vi "Periodic Tasks.vi"(8 "error in":errorcluster) -> (0 "error out":errorcluster)   [LabVIEW 2018]
doc: "This VI runs in parallel to other tasks. It can contain as many user-defined periodic loops as you need. These can carry out PID or other sorts of timed response."
uses:
  <vilib>/Rock Robotics/WPI/Joystick/WPI_JoystickDevRef.ctl
  <vilib>/Rock Robotics/WPI/Joystick/WPI_JoystickDeviceEnum.ctl
  <vilib>/Rock Robotics/WPI/RobotDrive/WPI_RobotDriveDevRef.ctl
  <vilib>/Rock Robotics/WPI/MotorControl/WPI_MotorControlDeviceRef.ctl
  <vilib>/Rock Robotics/WPI/MotorControl/WPI_MotorControlType.ctl
  <vilib>/Rock Robotics/SystemInterfaces/DIO/FPGA_DIOPWMChannel.ctl
  <vilib>/Rock Robotics/WPI/PWM/WPI_PWMDeadband.ctl
  <vilib>/Rock Robotics/SystemInterfaces/DIO/FPGA_DIOChannel.ctl
  <vilib>/Rock Robotics/WPI/Solenoid/WPI_SolenoidDevRef.ctl
  <vilib>/Rock Robotics/WPI/Solenoid/WPI_SolenoidChannel.ctl
  <vilib>/Rock Robotics/WPI/DigitalInput/WPI_DigitalInputDevRef.ctl
  Vision States.ctl
  <vilib>/Rock Robotics/WPI/DriverStation/WPI_DriverStationRobotMode2.ctl
  Hatch Retainer States.ctl
  HAB Bk Spd Motor States.ctl
  <vilib>/Rock Robotics/WPI/Solenoid/WPI_SolenoidValue.ctl
  <vilib>/Rock Robotics/WPI/ThirdParty/Phoenix-LabVIEW/Motor Controller/Controls/CTRE_Phoenix_MotorControl_ControlMode.ctl
  <vilib>/Rock Robotics/WPI/ThirdParty/Phoenix-LabVIEW/Motor Controller/Controls/CTRE_Phoenix_MotorControl_MotionProfileTrajectoryPoint.ctl
  <vilib>/Rock Robotics/WPI/Utilities/WPI_GetSetVariantRefNum.vi
  <vilib>/Rock Robotics/WPI/ThirdParty/Phoenix-LabVIEW/Motor Controller/Get/CTRE_Phoenix_MotorController_GetQuadratureData.vi
  Robot Global Data.vi
  <vilib>/addons/control/pid/pid.llb/PID (DBL).vi
  <vilib>/Rock Robotics/WPI/Solenoid/WPI_SolenoidSetEnum.vi
  <vilib>/Rock Robotics/Network Tables/NT Write Number.vi
  <vilib>/Rock Robotics/WPI/ThirdParty/Phoenix-LabVIEW/Motor Controller/Closed Loop/Motion Profile/CTRE_Phoenix_MotorControl_BufferedTrajectoryPointStream_WriteAll.vi
  <vilib>/Rock Robotics/Network Tables/NT Read Number.vi
  <vilib>/addons/control/pid/NI_PID_pid.lvlib
panel:
  in  "BkSpdAdjusterMotorDevRef":T1={"DeviceStatus"={"status"=FALSE, "code"=0, "source"=""}, "Type"=enum."PWM", "PWM"={"PWM Channel"=enum."Invalid", "DeadBand"={"Name"="", "maxPositivePwm"=0, "minPositivePwm"=0, "centerPwm"=0, "maxNegativePwm"=0, "minNegativePwm"=0, "angularRange"=0}}, "CAN"={"Device Number"=0, "SetOutput VI Ref"=variant(refnum<vi> refnum), "GetOutput VI Ref"=variant(refnum<vi> refnum), "Enable VI Ref"=variant(refnum<vi> refnum), "Disable VI Ref"=variant(refnum<vi> refnum), "Data"=variant}, "Invert"=FALSE, "DIO PWM"={"PWM \"Enable\" Channel"=enum."Invalid", "DIOChannel"=enum."Invalid", "PWM Rate"=0.0}}
  in  "HABAssisterSolenoidDevRef":T6={"DevStatus"={"status"=FALSE, "code"=0, "source"=""}, "Pneumatics Control Module"=0, "Forward Solenoid Channel"=enum."Invalid", "Reverse Solenoid Channel"=enum."Invalid"}
  out "Right Traj. Pts Array":dbl[][](array[numeric])
  out "Left Traj. Pts Array":dbl[][](array[numeric])
  in  "Back HAB 3 Limit Switch":T8={"DevStatus"={"status"=FALSE, "code"=0, "source"=""}, "DIO Channel"=enum."Invalid"}
  in  "Front HAB 3 Limit Switch":T8={"DevStatus"={"status"=FALSE, "code"=0, "source"=""}, "DIO Channel"=enum."Invalid"}
  in  "BottomRetainerSwitchDevRef":T8={"DevStatus"={"status"=FALSE, "code"=0, "source"=""}, "DIO Channel"=enum."Invalid"}
  in  "TopRetainerSwitchDevRef":T8={"DevStatus"={"status"=FALSE, "code"=0, "source"=""}, "DIO Channel"=enum."Invalid"}
  in  "HatchRetainerMotorDevRef":T1={"DeviceStatus"={"status"=FALSE, "code"=0, "source"=""}, "Type"=enum."PWM", "PWM"={"PWM Channel"=enum."Invalid", "DeadBand"={"Name"="", "maxPositivePwm"=0, "minPositivePwm"=0, "centerPwm"=0, "maxNegativePwm"=0, "minNegativePwm"=0, "angularRange"=0}}, "CAN"={"Device Number"=0, "SetOutput VI Ref"=variant(refnum<vi> refnum), "GetOutput VI Ref"=variant(refnum<vi> refnum), "Enable VI Ref"=variant(refnum<vi> refnum), "Disable VI Ref"=variant(refnum<vi> refnum), "Data"=variant}, "Invert"=FALSE, "DIO PWM"={"PWM \"Enable\" Channel"=enum."Invalid", "DIOChannel"=enum."Invalid", "PWM Rate"=0.0}}
  in  "HAB3BackSolenoidDevRef":T6={"DevStatus"={"status"=FALSE, "code"=0, "source"=""}, "Pneumatics Control Module"=0, "Forward Solenoid Channel"=enum."Invalid", "Reverse Solenoid Channel"=enum."Invalid"}
  in  "HAB3FrontSolenoidDevRef":T6={"DevStatus"={"status"=FALSE, "code"=0, "source"=""}, "Pneumatics Control Module"=0, "Forward Solenoid Channel"=enum."Invalid", "Reverse Solenoid Channel"=enum."Invalid"}
  in  "AuxJoystickDevRef":T9={"Device"=enum."USB 1"}
  in  "DriveJoystickDevRef":T9={"Device"=enum."USB 1"}
  in  "HAB3DriveModuleMotorDevRef":T1={"DeviceStatus"={"status"=FALSE, "code"=0, "source"=""}, "Type"=enum."PWM", "PWM"={"PWM Channel"=enum."Invalid", "DeadBand"={"Name"="", "maxPositivePwm"=0, "minPositivePwm"=0, "centerPwm"=0, "maxNegativePwm"=0, "minNegativePwm"=0, "angularRange"=0}}, "CAN"={"Device Number"=0, "SetOutput VI Ref"=variant(refnum<vi> refnum), "GetOutput VI Ref"=variant(refnum<vi> refnum), "Enable VI Ref"=variant(refnum<vi> refnum), "Disable VI Ref"=variant(refnum<vi> refnum), "Data"=variant}, "Invert"=FALSE, "DIO PWM"={"PWM \"Enable\" Channel"=enum."Invalid", "DIOChannel"=enum."Invalid", "PWM Rate"=0.0}}
  in  "LifterSolenoidDevRef":T6={"DevStatus"={"status"=FALSE, "code"=0, "source"=""}, "Pneumatics Control Module"=0, "Forward Solenoid Channel"=enum."Invalid", "Reverse Solenoid Channel"=enum."Invalid"}
  in  "DriveJoystickDevRef":T9={"Device"=enum."USB 1"}
  in  "HatchCollectorMotorDevRef":T1={"DeviceStatus"={"status"=FALSE, "code"=0, "source"=""}, "Type"=enum."PWM", "PWM"={"PWM Channel"=enum."Invalid", "DeadBand"={"Name"="", "maxPositivePwm"=0, "minPositivePwm"=0, "centerPwm"=0, "maxNegativePwm"=0, "minNegativePwm"=0, "angularRange"=0}}, "CAN"={"Device Number"=0, "SetOutput VI Ref"=variant(refnum<vi> refnum), "GetOutput VI Ref"=variant(refnum<vi> refnum), "Enable VI Ref"=variant(refnum<vi> refnum), "Disable VI Ref"=variant(refnum<vi> refnum), "Data"=variant}, "Invert"=FALSE, "DIO PWM"={"PWM \"Enable\" Channel"=enum."Invalid", "DIOChannel"=enum."Invalid", "PWM Rate"=0.0}}
  in  "AuxJoystickDevRef":T9
  in  "RetainerSolenoidDevRef":T6={"DevStatus"={"status"=FALSE, "code"=0, "source"=""}, "Pneumatics Control Module"=0, "Forward Solenoid Channel"=enum."Invalid", "Reverse Solenoid Channel"=enum."Invalid"}
  in  "KickerSolenoidDevRef":T6={"DevStatus"={"status"=FALSE, "code"=0, "source"=""}, "Pneumatics Control Module"=0, "Forward Solenoid Channel"=enum."Invalid", "Reverse Solenoid Channel"=enum."Invalid"}
  in  "Drive Motors":T11={"DevStatus"={"status"=FALSE, "code"=0, "source"=""}, "Motors[]"=[], "Square Inputs"=FALSE, "Max Output"=1.0}
  in  "AuxJoystickDevRef":T9={"Device"=enum."USB 1"}
  in  "DriveJoystickDevRef":T9
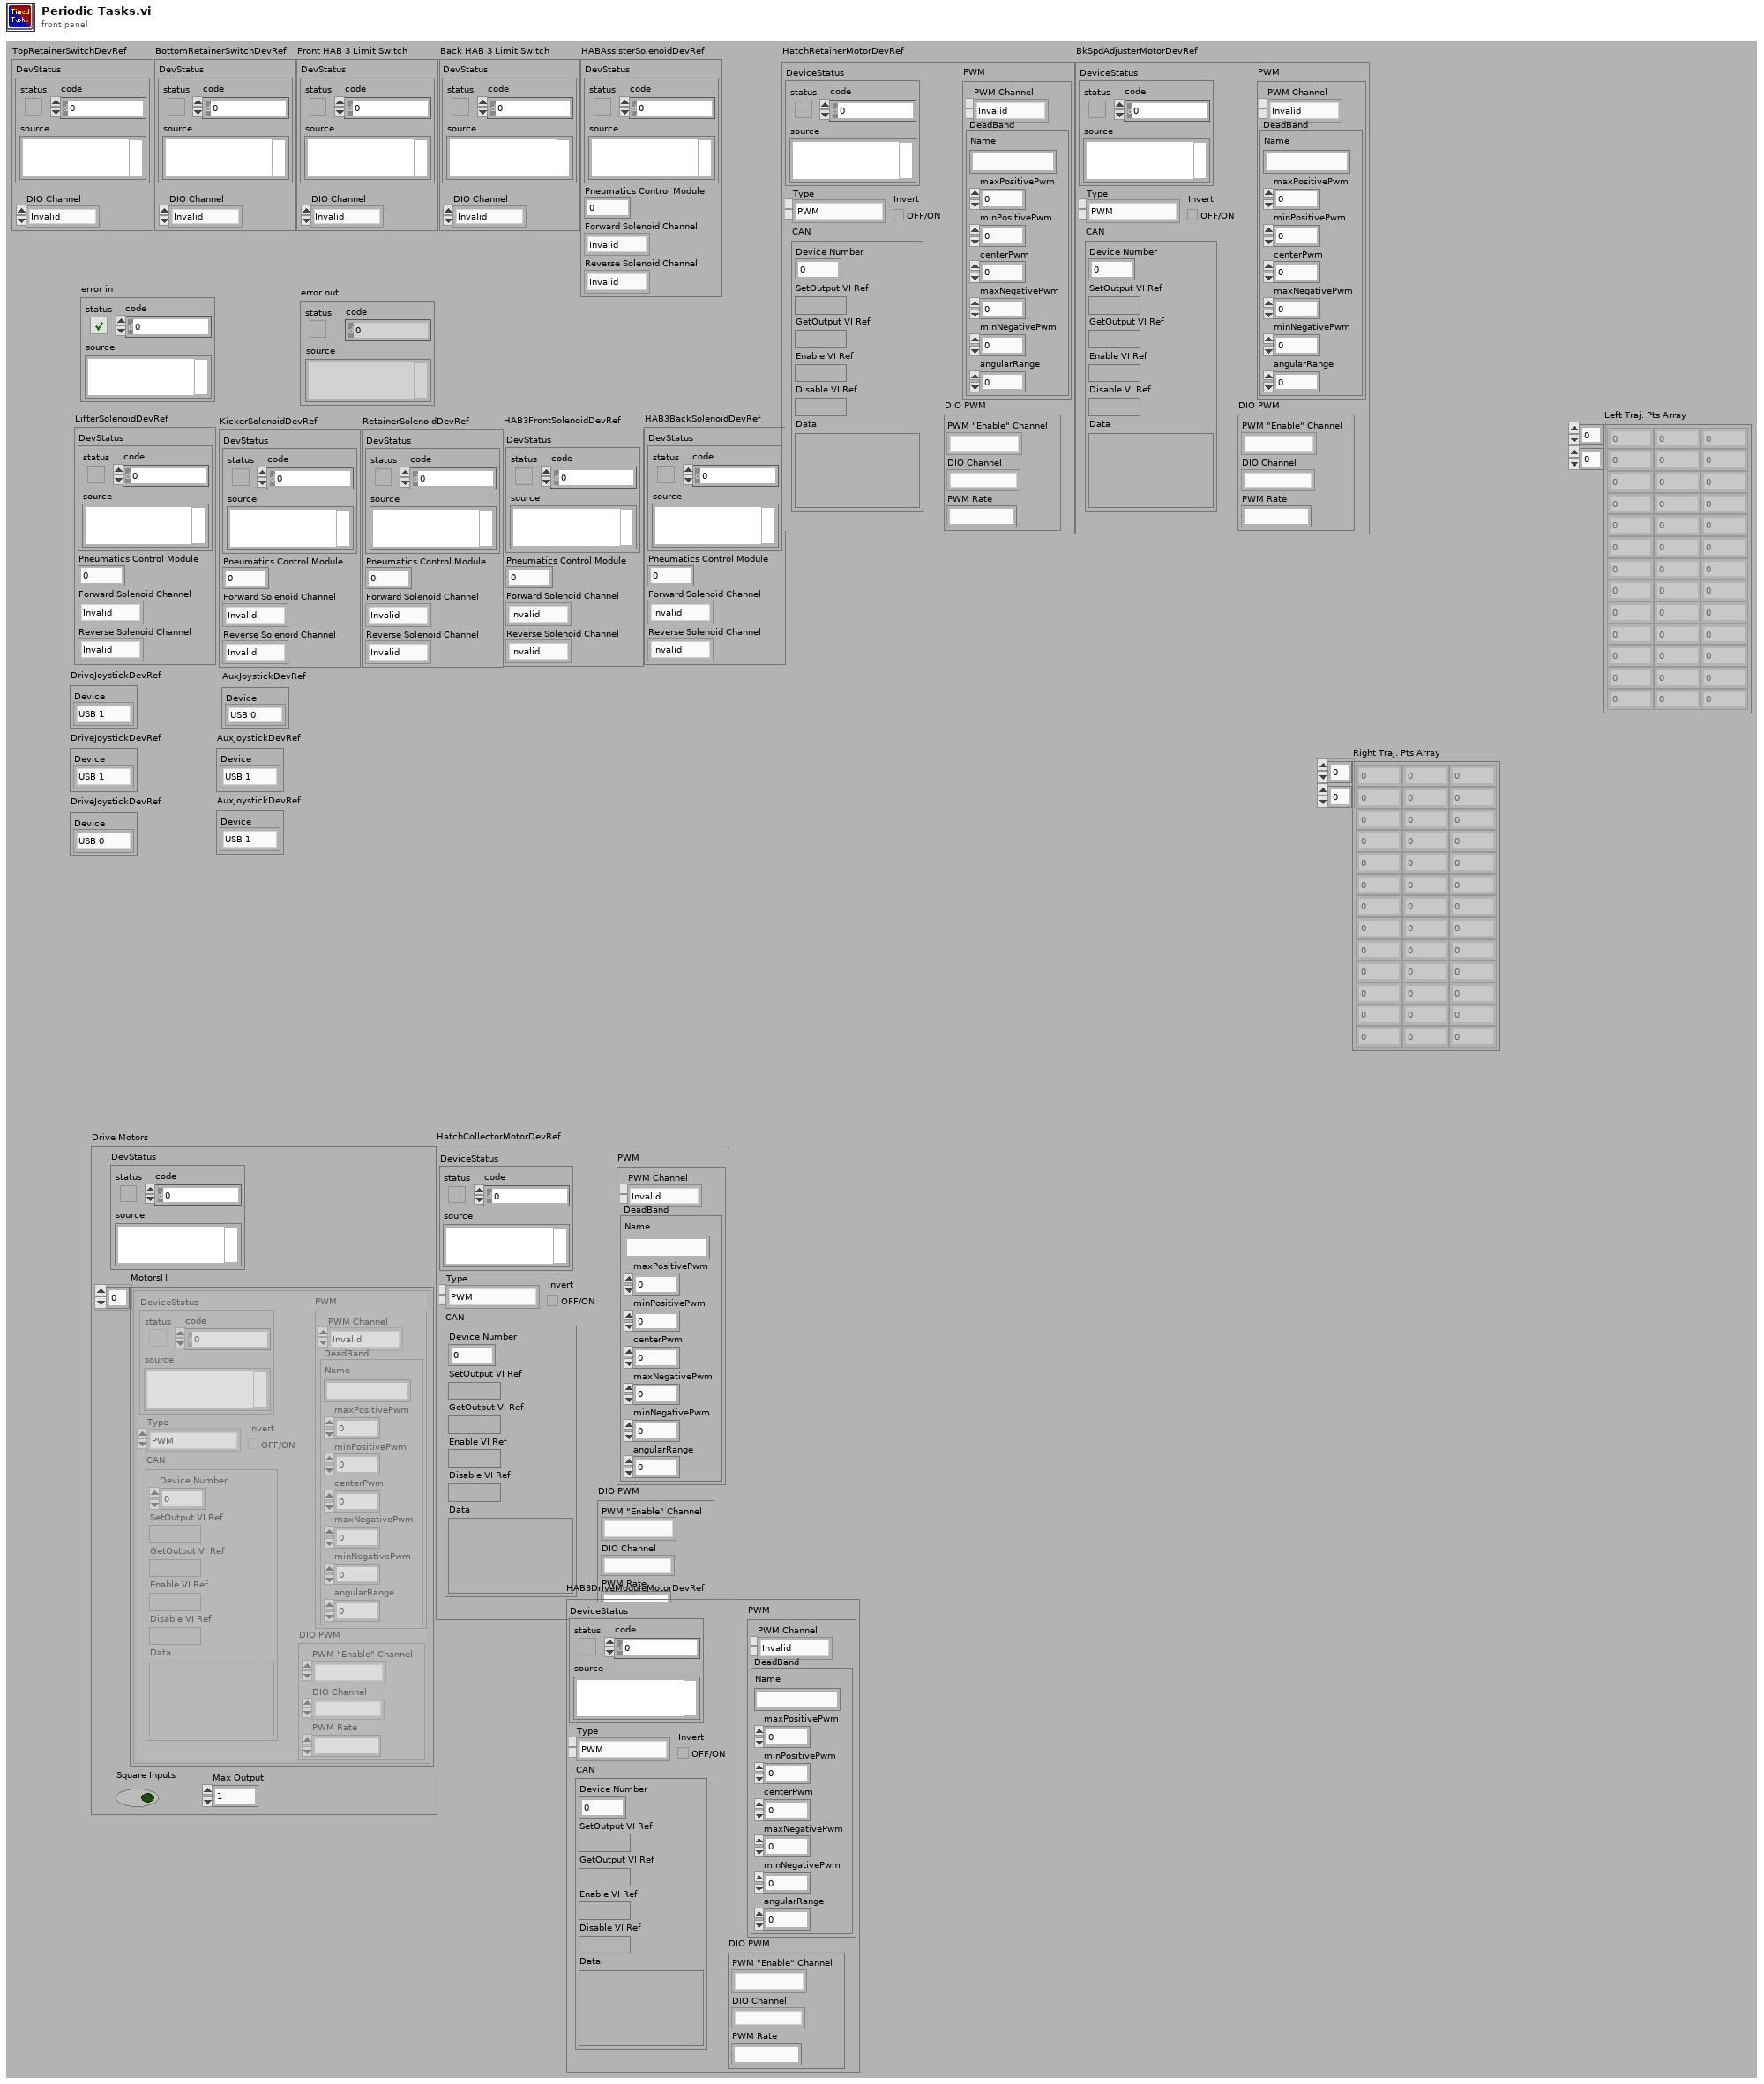
[diagram p1: front panel]
types:
  T1 = typedef "WPI_MotorControlDeviceRef.ctl" = cluster{"DeviceStatus":errorcluster, "Type":T2, "PWM":cluster{"PWM Channel":T3, "DeadBand":T4}, "CAN":cluster{"Device Number":u8, "SetOutput VI Ref":variant, "GetOutput VI Ref":variant, "Enable VI Ref":variant, "Disable VI Ref":variant, "Data":variant}, "Invert":bool, "DIO PWM":cluster{"PWM \"Enable\" Channel":T3, "DIOChannel":T5, "PWM Rate":dbl}}
  T2 = typedef "WPI_MotorControlType.ctl" = enum16{"PWM", "CAN", "DIO PWM"}
  T3 = typedef "FPGA_DIOPWMChannel.ctl" = enum8{"PWM 0", "PWM 1", "PWM 2", "PWM 3", "PWM 4", "PWM 5", "PWM 6", "PWM 7", "PWM 8", "PWM 9", "PWM MXP 0", "PWM MXP 1", "PWM MXP 2", "PWM MXP 3", "PWM MXP 4", "PWM MXP 5", "PWM MXP 6", "PWM MXP 7", "PWM MXP 8", "PWM MXP 9", "Invalid"}
  T4 = typedef "WPI_PWMDeadband.ctl" = cluster{"Name":string, "maxPositivePwm":i32, "minPositivePwm":i32, "centerPwm":i32, "maxNegativePwm":i32, "minNegativePwm":i32, "angularRange":u16}
  T5 = typedef "FPGA_DIOChannel.ctl" = enum8{"DIO 0", "DIO 1", "DIO 2", "DIO 3", "DIO 4", "DIO 5", "DIO 6", "DIO 7", "DIO 8", "DIO 9", "DIO MXP 0", "DIO MXP 1", "DIO MXP 2", "DIO MXP 3", "DIO MXP 4", "DIO MXP 5", "DIO MXP 6", "DIO MXP 7", "DIO MXP 8", "DIO MXP 9", "DIO MXP 10", "DIO MXP 11", "DIO MXP 12", "DIO MXP 13", "DIO MXP 14", "DIO MXP 15", "SPI Port CS1", "SPI Port CS2", "SPI Port CS3", "SPI Port MISO", "SPI Port MOSI", "Invalid"}
  T6 = typedef "WPI_SolenoidDevRef.ctl" = cluster{"DevStatus":errorcluster, "Pneumatics Control Module":u8, "Forward Solenoid Channel":T7, "Reverse Solenoid Channel":T7}
  T7 = typedef "WPI_SolenoidChannel.ctl" = enum8{"Solenoid 0", "Solenoid 1", "Solenoid 2", "Solenoid 3", "Solenoid 4", "Solenoid 5", "Solenoid 6", "Solenoid 7", "Invalid"}
  T8 = typedef "WPI_DigitalInputDevRef.ctl" = cluster{"DevStatus":errorcluster, "DIO Channel":T5}
  T9 = typedef "WPI_JoystickDevRef.ctl" = cluster{"Device":T10}
  T10 = typedef "WPI_JoystickDeviceEnum.ctl" = enum16{"USB 0", "USB 1", "USB 2", "USB 3", "USB 4", "USB 5"}
  T11 = typedef "WPI_RobotDriveDevRef.ctl" = cluster{"DevStatus":errorcluster, "Motors[]":T1[], "Square Inputs":bool, "Max Output":dbl}
  T12 = typedef "HAB Bk Spd Motor States.ctl" = enum16{"Fully Up", "Going Down", "Fully Down", "Going Up"}
  T13 = typedef "Hatch Retainer States.ctl" = enum16{"Fully Down", "Going Up", "Fully Up", "Going Down"}
  T14 = cluster{"X Button":i32, "A Button":i32, "B Button":i32, "Y Button":i32, "LB Button":i32, "RB Button":i32, "LT Button":i32, "RT Button":i32, "BACK Button":i32, "START Button":i32, "LJ Click Button":i32, "RJ Click Button":i32}
  T15 = cluster{"Left X":i32, "Left Y":i32, "Right X":i32, "Right Y":i32}
  T16 = typedef "WPI_DriverStationRobotMode2.ctl" = enum16{"Autonomous Disabled", "Autonomous Enabled", "Teleop Disabled", "Teleop Enabled", "Disconnected", "Finish", "Test Disabled", "Test Enabled", "Emergency Stopped"}
  T17 = cluster{"offsetAngle H":dbl, "offsetAngle V":dbl, "area":dbl, "skew":dbl, "shortest side (pxls)":dbl, "longest side (pxls)":dbl}
  T18 = typedef "Vision States.ctl" = enum16{"Ready", "Forward Until Target at Edge", "Vision Track"}
  T19 = cluster{"A Button":i32, "B Button":i32, "X Button":i32, "Y Button":i32, "LB Button":i32, "RB Button":i32, "BACK Button":i32, "START Button":i32, "LJ Click Button":i32, "RJ Click Button":i32}
  T20 = typedef "WPI_GyroDevRef.ctl" = cluster{"DevStatus":errorcluster, "Analog Channel":T21, "Gain (VoltsPerDegree/Second)":dbl, "Gyro Type":enum16{"Analog", "XRS450"}, "Handle":i32, "SPI Bus":T22, "Device Found":bool, "Sample Rate":dbl, "Calibrate On Open":bool, "Offset":dbl}
  T21 = typedef "FPGA_AIChannel.ctl" = enum8{"AI 0", "AI 1", "AI 2", "AI 3", "AI MXP 0", "AI MXP 1", "AI MXP 2", "AI MXP 3", "Invalid"}
  T22 = typedef "spi_bus.ctl" = enum16{"SPI On-Board, CS0", "SPI On-Board, CS1", "SPI On-Board, CS2", "SPI On-Board, CS3", "SPI MXP", "Invalid"}
  T23 = cluster{"DriveJoystickDevRef":T9, "AuxJoystickDevRef":T9, "Drive Axes":dbl[], "Drive Buttons":bool[], "Drive POVs":i16[], "Aux Axes":dbl[], "Aux Buttons":bool[], "Aux POVs":i16[], "Robot Mode":T16, "Drive Motors":T11, "Drive Joystick Indexes":cluster{"Left X":i32, "Left Y":i32, "Right X":i32, "Right Y":i32}, "Drive Button Indexes":cluster{"A Button":i32, "B Button":i32, "X Button":i32, "Y Button":i32, "LB Button":i32, "RB Button":i32, "BACK Button":i32, "START Button":i32, "LJ Click Button":i32, "RJ Click Button":i32}, "Joystick VS Vision Latch":bool, "Vision States":T18, "limelight":cluster{"offsetAngle H":dbl, "offsetAngle V":dbl, "area":dbl, "skew":dbl, "shortest side (pxls)":dbl, "longest side (pxls)":dbl}, "Vision Track Mode Override":bool, "T = Motion Profile, F = Percent Output":bool}
  T24 = cluster{"TopRetainerSwitchDevRef":T8, "BottomRetainerSwitchDevRef":T8, "HatchRetainerMotorDevRef":T1, "LifterSolenoidDevRef":T6, "DriveJoystickDevRef":T9, "KickerSolenoidDevRef":T6, "RetainerSolenoidDevRef":T6, "AuxJoystickDevRef":T9, "HatchCollectorMotorDevRef":T1, "Drive Axes":dbl[], "Drive Buttons":bool[], "Drive POVs":i16[], "Aux Axes":dbl[], "Aux Buttons":bool[], "Aux POVs":i16[], "Robot Mode":T16, "Aux Joystick Indexes":cluster{"Left X":i32, "Left Y":i32, "Right X":i32, "Right Y":i32}, "Aux Button Indexes":cluster{"X Button":i32, "A Button":i32, "B Button":i32, "Y Button":i32, "LB Button":i32, "RB Button":i32, "LT Button":i32, "RT Button":i32, "BACK Button":i32, "START Button":i32, "LJ Click Button":i32, "RJ Click Button":i32}, "Hatch Retainer Move Up/Down":bool, "Hatch Collector Actual Angle":dbl, "Hatch Collector Wanted Angle":dbl, "Hatch Retainer States":T13}
  T25 = cluster{"BkSpdAdjusterMotorDevRef":T1, "HABAssisterSolenoidDevRef":T6, "Back HAB 3 Limit Switch":T8, "Front HAB 3 Limit Switch":T8, "HAB3DriveModuleMotorDevRef":T1, "DriveJoystickDevRef":T9, "AuxJoystickDevRef":T9, "HAB3FrontSolenoidDevRef":T6, "HAB3BackSolenoidDevRef":T6, "Drive Axes":dbl[], "Drive Buttons":bool[], "Drive POVs":i16[], "Aux Axes":dbl[], "Aux Buttons":bool[], "Aux POVs":i16[], "Robot Mode":T16, "Aux Joystick Indexes":cluster{"Left X":i32, "Left Y":i32, "Right X":i32, "Right Y":i32}, "Aux Button Indexes":cluster{"X Button":i32, "A Button":i32, "B Button":i32, "Y Button":i32, "LB Button":i32, "RB Button":i32, "LT Button":i32, "RT Button":i32, "BACK Button":i32, "START Button":i32, "LJ Click Button":i32, "RJ Click Button":i32}, "Front Cylinders Latch":bool, "Back Cylinders Latch":bool, "Yaw":dbl, "Pitch":dbl, "Roll":dbl, "HAB Bk Spd Motor States":T12}
  T26 = typedef "WPI_SolenoidValue.ctl" = enum16{"Off", "On", "Forward", "Reverse"}
  T27 = cluster{"proportional gain (Kc)":dbl, "integral time (Ti, min)":dbl, "derivative time (Td, min)":dbl}
  T28 = typedef "Which Robot Enum.ctl" = enum16{"Competition Bot", "Practice Bot", "Code Bot"}
  T29 = typedef "CTRE_Phoenix_MotorControl_ControlMode.ctl" = u16
  T30 = cluster{"Yaw":dbl, "Roll":dbl, "Pitch":dbl, "Heading":dbl, "Fused Heading":dbl}
  T31 = typedef "CTRE_Phoenix_MotorControl_MotionProfileTrajectoryPoint.ctl" = cluster{"Position":dbl, "Velocity":dbl, "Arbitrary Feed Forward":dbl, "Auxiliary Position":dbl, "Auxiliary Velocity":dbl, "Auxiliary Arbitrary Feed Forward":dbl, "Profile Slot Select":i32, "Auxiliary Profile Slot Select":i32, "isLastPoint?":bool, "Zero Position?":bool, "durationMs":u32, "Use Aux PID?":bool}
  T32 = typedef "CTRE_Phoenix_MotorControl_BufferedTrajectoryPointStream_DeviceRef.ctl" = cluster{"Handle":u64, "Library Path":path}
  T33 = cluster{"DriveJoystickDevRef":T9, "AuxJoystickDevRef":T9, "Drive Axes":dbl[], "Drive Buttons":bool[], "Drive POVs":i16[], "Aux Axes":dbl[], "Aux Buttons":bool[], "Aux POVs":i16[], "Robot Mode":T16, "Drive Motors":T11, "Drive Joystick Indexes":cluster{"Left X":i32, "Left Y":i32, "Right X":i32, "Right Y":i32}, "Drive Button Indexes":cluster{"A Button":i32, "B Button":i32, "X Button":i32, "Y Button":i32, "LB Button":i32, "RB Button":i32, "BACK Button":i32, "START Button":i32, "LJ Click Button":i32, "RJ Click Button":i32}, "Joystick VS Vision Latch":bool, "Vision States":T18, "limelight":cluster{"offsetAngle H":dbl, "offsetAngle V":dbl, "area":dbl, "skew":dbl, "shortest side (pxls)":dbl, "longest side (pxls)":dbl}, "Vision Track Mode Override":bool, "T = Motion Profile, F = Percent Output (Latch)":bool}
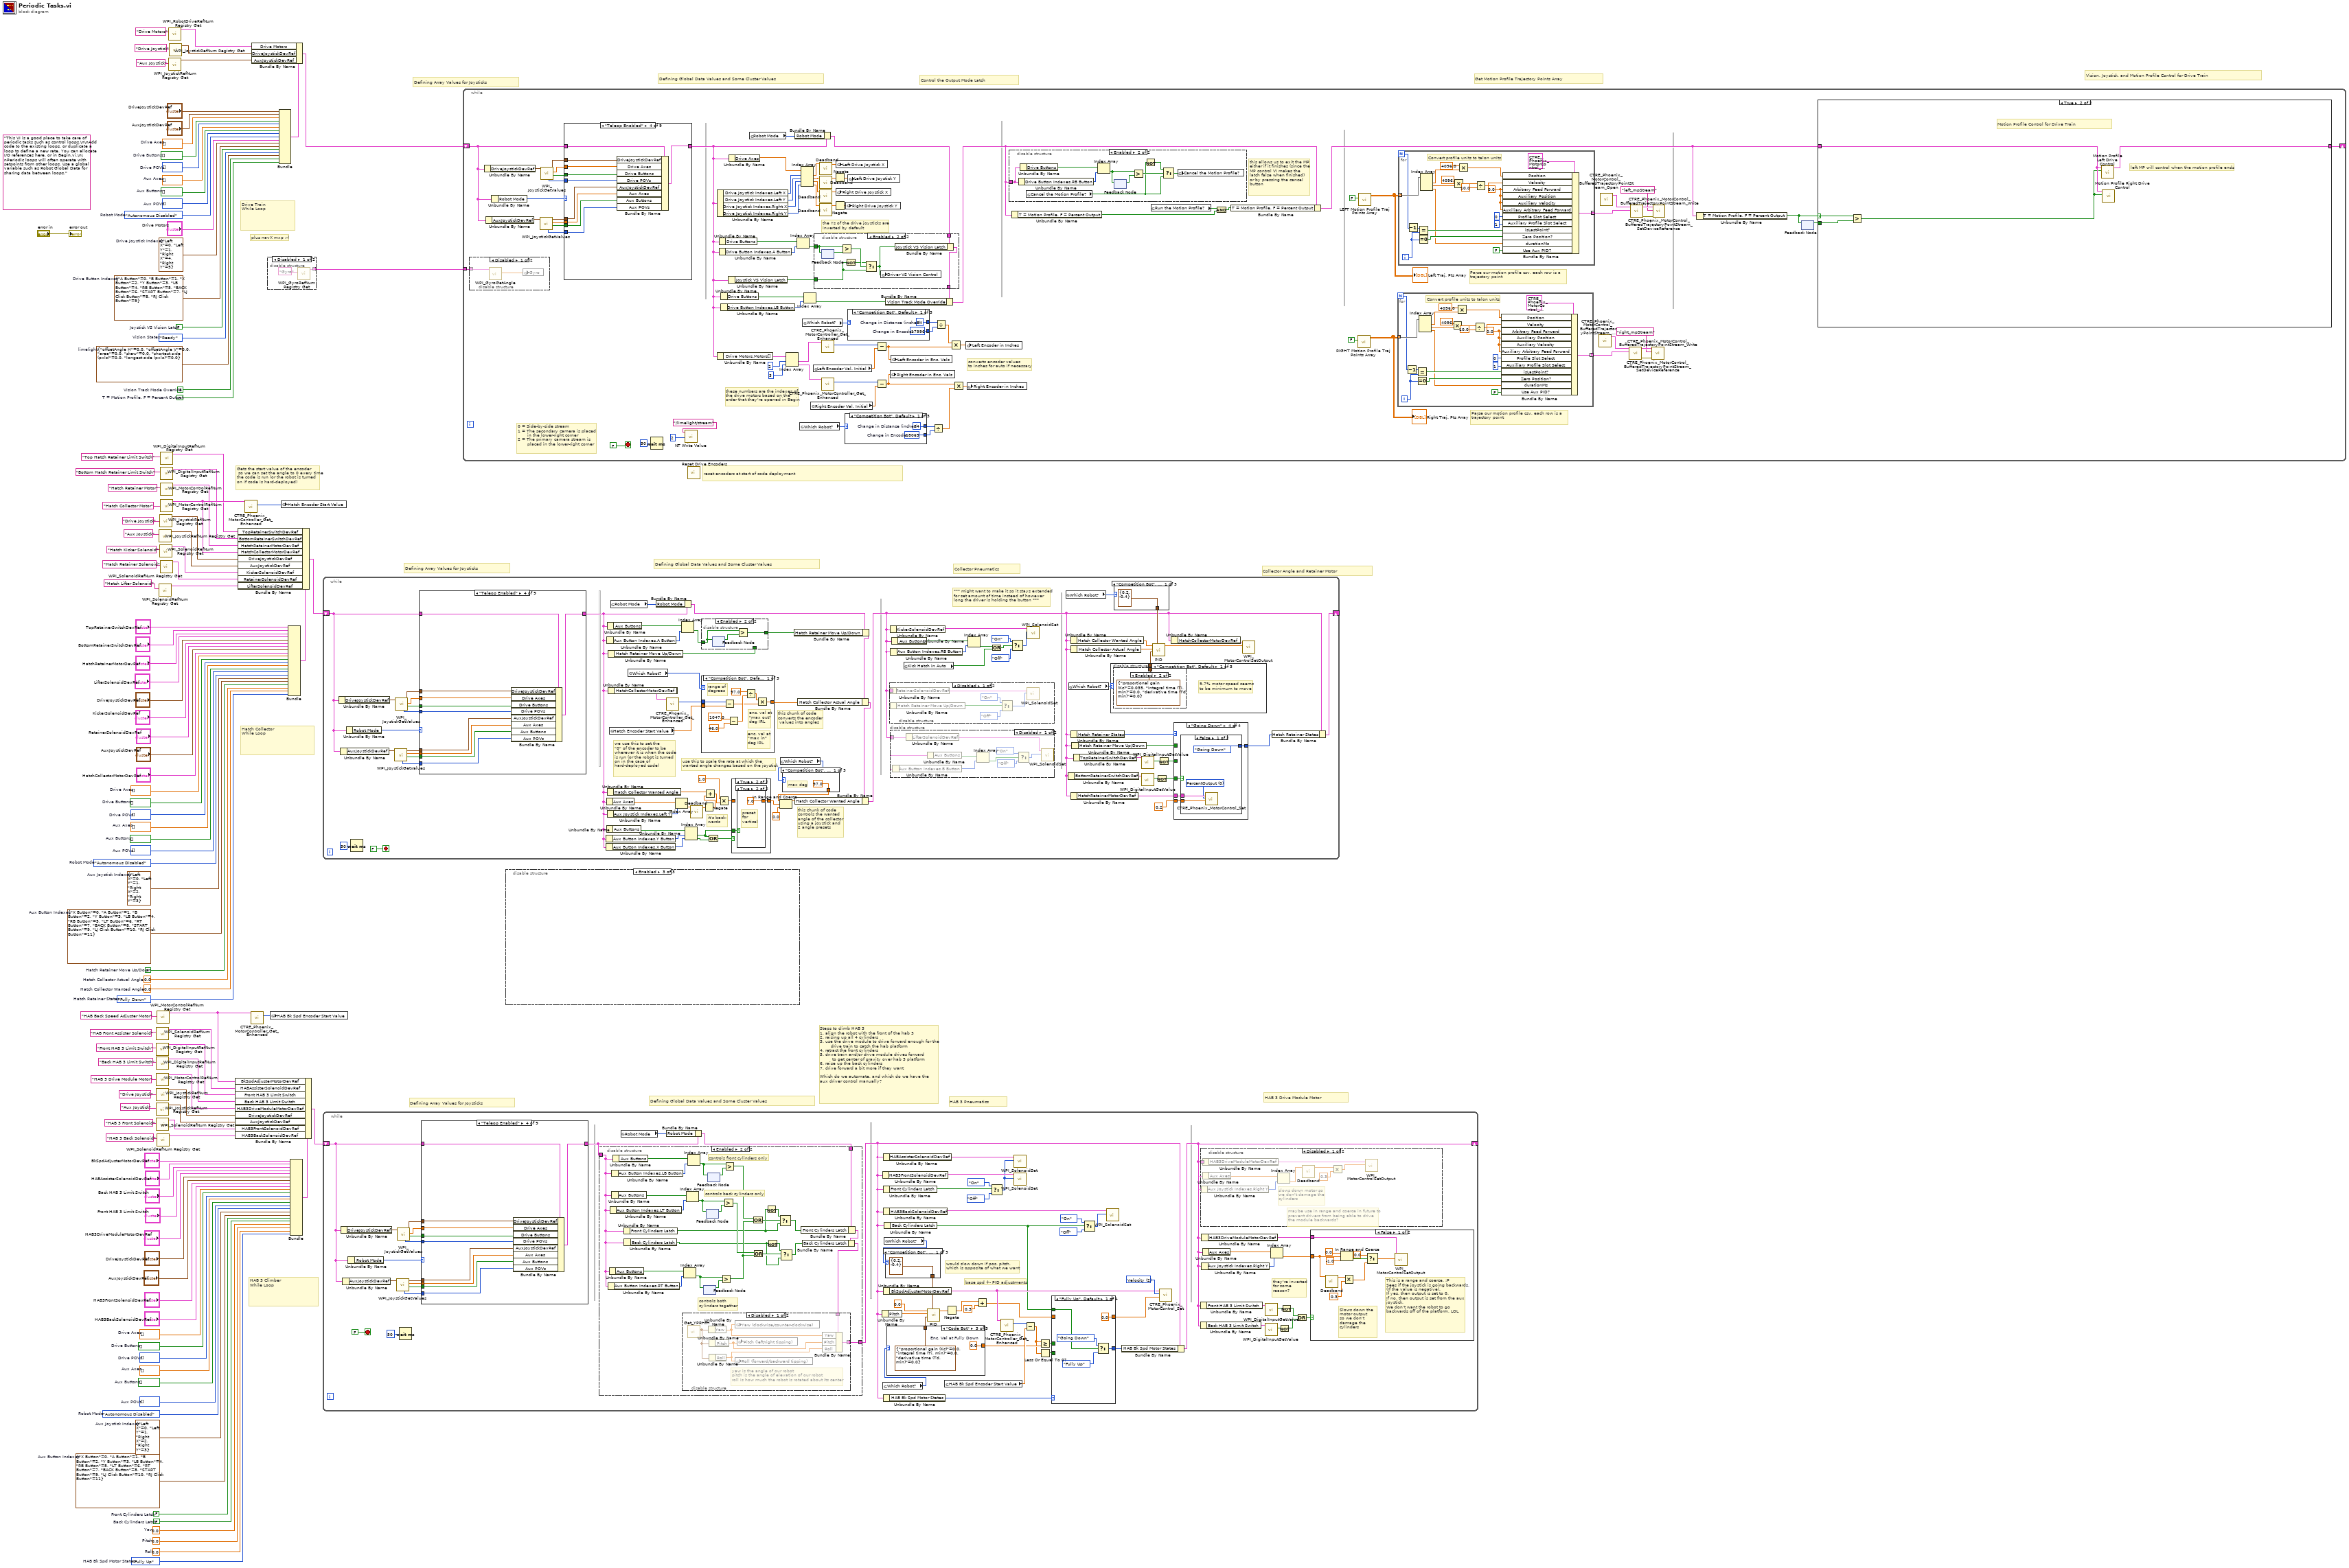
[diagram p0: block diagram]
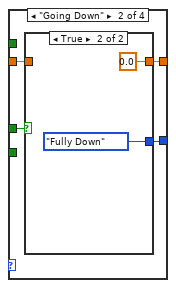
[diagram p5: hidden frame]
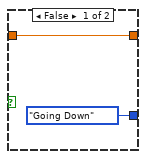
[diagram p6: hidden frame]
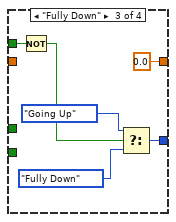
[diagram p7: hidden frame]
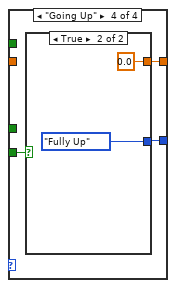
[diagram p8: hidden frame]
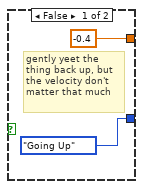
[diagram p9: hidden frame]
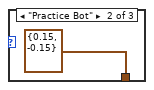
[diagram p10: hidden frame]
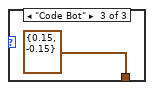
[diagram p11: hidden frame]
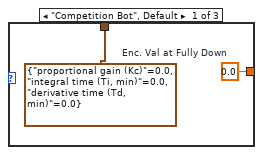
[diagram p12: hidden frame]
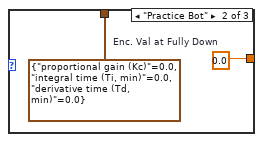
[diagram p13: hidden frame]
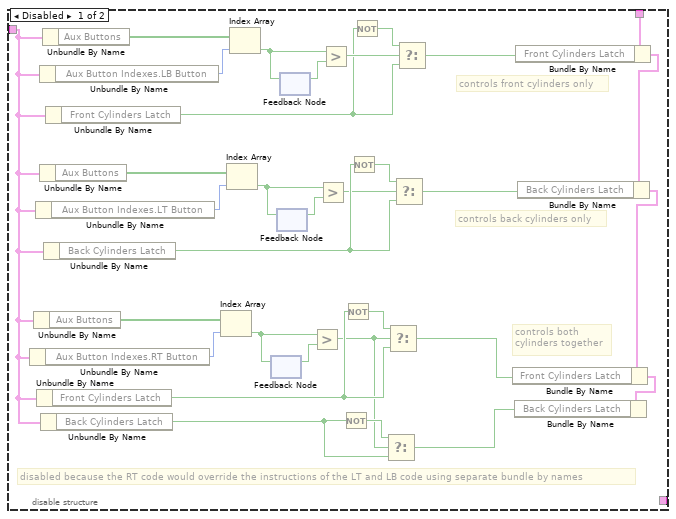
[diagram p14: hidden frame]
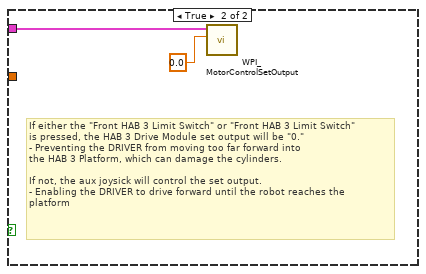
[diagram p17: hidden frame]
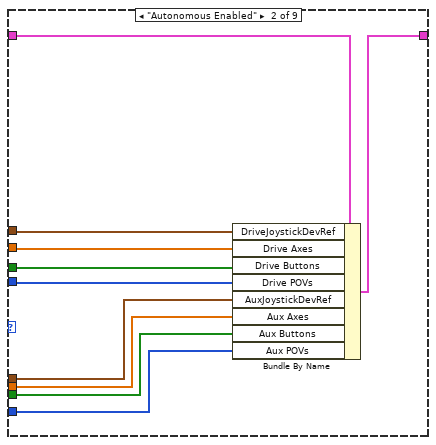
[diagram p19: hidden frame]
diagram:
  w1 = HAB_Bk_Spd_Motor_States."Fully Up"  # HAB Bk Spd Motor States
  w6 = 0.0  # Roll
  w7 = 0.0  # Pitch
  w8 = 0.0  # Yaw
  w18 = Hatch_Retainer_States."Fully Down"  # Hatch Retainer States
  w28 = FALSE  # T = Motion Profile, F = Percent Output
  w30 = 0.0  # Hatch Collector Wanted Angle
  w31 = FALSE  # Back Cylinders Latch
  w32 = FALSE  # Front Cylinders Latch
  w33 = T14 {"X Button"=0, "A Button"=1, "B Button"=2, "Y Button"=3, "LB Button"=4, "RB Button"=5, "LT Button"=6, "RT Button"=7, "BACK Button"=8, "START Button"=9, "LJ Click Button"=10, "RJ Click Button"=11}  # Aux Button Indexes
  w34 = T15 {"Left X"=0, "Left Y"=1, "Right X"=2, "Right Y"=3}  # Aux Joystick Indexes
  w35 = WPI_DriverStationRobotMode2."Autonomous Disabled"  # Robot Mode
  w36 = i16[] []  # Aux POVs
  w37 = bool[] []  # Aux Buttons
  w38 = dbl[] []  # Aux Axes
  w39 = i16[] []  # Drive POVs
  w40 = bool[] []  # Drive Buttons
  w41 = dbl[] []  # Drive Axes
  w64 = 0.0  # Hatch Collector Actual Angle
  w65 = FALSE  # Hatch Retainer Move Up/Down
  w66 = T14 {"X Button"=0, "A Button"=1, "B Button"=2, "Y Button"=3, "LB Button"=4, "RB Button"=5, "LT Button"=6, "RT Button"=7, "BACK Button"=8, "START Button"=9, "LJ Click Button"=10, "RJ Click Button"=11}  # Aux Button Indexes
  w67 = T15 {"Left X"=0, "Left Y"=1, "Right X"=2, "Right Y"=3}  # Aux Joystick Indexes
  w71 = WPI_DriverStationRobotMode2."Autonomous Disabled"  # Robot Mode
  w72 = i16[] []  # Aux POVs
  w73 = bool[] []  # Aux Buttons
  w74 = dbl[] []  # Aux Axes
  w75 = i16[] []  # Drive POVs
  w76 = bool[] []  # Drive Buttons
  w77 = dbl[] []  # Drive Axes
  w91 = FALSE  # Vision Track Mode Override
  w92 = T17 {"offsetAngle H"=0.0, "offsetAngle V"=0.0, "area"=0.0, "skew"=0.0, "shortest side (pxls)"=0.0, "longest side (pxls)"=0.0}  # limelight
  w93 = Vision_States."Ready"  # Vision States
  w94 = FALSE  # Joystick VS Vision Latch
  w95 = T19 {"A Button"=0, "B Button"=1, "X Button"=2, "Y Button"=3, "LB Button"=4, "RB Button"=5, "BACK Button"=6, "START Button"=7, "LJ Click Button"=8, "RJ Click Button"=9}  # Drive Button Indexes
  w97 = T15 {"Left X"=0, "Left Y"=1, "Right X"=4, "Right Y"=5}  # Drive Joystick Indexes
  w102 = i16[] []  # Aux POVs
  w103 = bool[] []  # Aux Buttons
  w104 = dbl[] []  # Aux Axes
  w101 = WPI_DriverStationRobotMode2."Autonomous Disabled"  # Robot Mode
  w105 = i16[] []  # Drive POVs
  w106 = bool[] []  # Drive Buttons
  w107 = dbl[] []  # Drive Axes
  (unwired) "This VI is a good place to take care of periodic tasks such as control loops.\n\nAdd code to the existing loops, or duplicate a loop to define a new rate. You can allocate I/O references here, or in Begin.vi.\n\nPeriodic loops will often operate with setpoints from other loops. Use a global variable such as Robot Global Data for sharing data between loops."
  # "reset encoders at start of code deployment"
  # "Get Motion Profile Trajectory Points Array"
  # "Control the Output Mode Latch"
  # "plus navX mxp :-)"
  # "HAB 3 Drive Module Motor"
  # "HAB 3 Pneumatics"
  # "Steps to climb HAB 3\n1. align the robot with the front of the hab 3\n2. raising up all 4 cylinders\n3. use the drive module to drive forward enough for the \n        drive train to catch the hab platform\n4. retract the front cylinders\n5. drive train and/or drive module drives forward \n         to get center of gravity over hab 3 platform\n6. raise up the back cylinders\n7. drive forward a bit more if they want\n\nWhich do we automate, and which do we have the \naux driver control manually?"
  # "Defining Global Data Values and Some Cluster Values"
  # "Defining Array Values for Joysticks"
  # "Gets the start value of the encoder\n so we can set the angle to 0 every time\nthe code is run (or the robot is turned\non if code is hard-deployed)"
  # "Collector Angle and Retainer Motor"
  # "Collector Pneumatics"
  # "Defining Global Data Values and Some Cluster Values"
  # "Defining Array Values for Joysticks"
  # "HAB 3 Climber\nWhile Loop"
  # "Hatch Collector\nWhile Loop"
  # "Drive Train\nWhile Loop"
  # "Vision, Joystick, and Motion Profile Control for Drive Train"
  # "Defining Array Values for Joysticks"
  # "Defining Global Data Values and Some Cluster Values"
  n1 = call <vilib>:"WPI_DigitalInputRefNum Registry Get.vi"("refnum name"="Front HAB 3 Limit Switch") -> ("DigitalInputDevRef"=w13:T8)  [unwired: 9 in, 1 out]
  n2 = call <vilib>:"WPI_JoystickRefNum Registry Get.vi"("refnum name"="Aux Joystick") -> ("JoystickDevRef"=w45:T9)  [unwired: 9 in, 1 out]
  n3 = call <vilib>:"WPI_SolenoidRefNum Registry Get.vi"("refnum name"="HAB Front Assister Solenoid") -> ("SolenoidDevRef"=w9:T6)  [unwired: 9 in, 1 out]
  n4 = call <vilib>:"WPI_DigitalInputRefNum Registry Get.vi"("refnum name"="Back HAB 3 Limit Switch") -> ("DigitalInputDevRef"=w12:T8)  [unwired: 9 in, 1 out]
  n5 = call <vilib>:"WPI_MotorControlRefNum Registry Get.vi"("refnum name"="HAB 3 Drive Module Motor") -> ("MotorControlDevRef"=w43:T1)  [unwired: 9 in, 1 out]
  n6 = call <vilib>:"WPI_JoystickRefNum Registry Get.vi"("refnum name"="Drive Joystick") -> ("JoystickDevRef"=w44:T9)  [unwired: 9 in, 1 out]
  n7 = call <vilib>:"WPI_SolenoidRefNum Registry Get.vi"("refnum name"="HAB 3 Front Solenoid") -> ("SolenoidDevRef"=w46:T6)  [unwired: 9 in, 1 out]
  n8 = call <vilib>:"WPI_MotorControlRefNum Registry Get.vi"("refnum name"="HAB Back Speed Adjuster Motor") -> ("MotorControlDevRef"=w2:T1)  [unwired: 9 in, 1 out]
  n9 = call <vilib>:"WPI_SolenoidRefNum Registry Get.vi"("refnum name"="HAB 3 Back Solenoid") -> ("SolenoidDevRef"=w47:T6)  [unwired: 9 in, 1 out]
  n10 = call <vilib>:"WPI_SolenoidRefNum Registry Get.vi"("refnum name"="Hatch Lifter Solenoid") -> ("SolenoidDevRef"=w60:T6)  [unwired: 9 in, 1 out]
  n11 = call <vilib>:"WPI_JoystickRefNum Registry Get.vi"("refnum name"="Aux Joystick") -> ("JoystickDevRef"=w82:T9)  [unwired: 9 in, 1 out]
  n12 = call <vilib>:"WPI_JoystickRefNum Registry Get.vi"("refnum name"="Drive Joystick") -> ("JoystickDevRef"=w68:T9)  [unwired: 9 in, 1 out]
  n13 = call <vilib>:"WPI_SolenoidRefNum Registry Get.vi"("refnum name"="Hatch Kicker Solenoid") -> ("SolenoidDevRef"=w85:T6)  [unwired: 9 in, 1 out]
  n14 = call <vilib>:"WPI_SolenoidRefNum Registry Get.vi"("refnum name"="Hatch Retainer Solenoid") -> ("SolenoidDevRef"=w84:T6)  [unwired: 9 in, 1 out]
  n15 = call <vilib>:"WPI_DigitalInputRefNum Registry Get.vi"("refnum name"="Top Hatch Retainer Limit Switch") -> ("DigitalInputDevRef"=w19:T8)  [unwired: 9 in, 1 out]
  n16 = call <vilib>:"WPI_DigitalInputRefNum Registry Get.vi"("refnum name"="Bottom Hatch Retainer Limit Switch") -> ("DigitalInputDevRef"=w20:T8)  [unwired: 9 in, 1 out]
  n17 = call <vilib>:"WPI_MotorControlRefNum Registry Get.vi"("refnum name"="Hatch Retainer Motor") -> ("MotorControlDevRef"=w25:T1)  [unwired: 9 in, 1 out]
  n18 = call <vilib>:"WPI_MotorControlRefNum Registry Get.vi"("refnum name"="Hatch Collector Motor") -> ("MotorControlDevRef"=w63:T1)  [unwired: 9 in, 1 out]
  n19 = call <vilib>:"WPI_RobotDriveRefNum Registry Get.vi"("refnum name"="Drive Motors") -> ("RobotDriveDevRef"=w99:T11)  [unwired: 9 in, 1 out]
  n20 = call <vilib>:"WPI_JoystickRefNum Registry Get.vi"("refnum name"="Aux Joystick") -> ("JoystickDevRef"=w109:T9)  [unwired: 9 in, 1 out]
  n21 = call <vilib>:"WPI_JoystickRefNum Registry Get.vi"("refnum name"="Drive Joystick") -> ("JoystickDevRef"=w110:T9)  [unwired: 9 in, 1 out]
  n22 = call-poly <vilib>:"CTRE_Phoenix_MotorController_Get_Enhanced.vi"("PhoenixMotorControlDevRef"=w63) -> ("Quadrature Position"=w62:i32)  [unwired: 11 in, 3 out]
  n23 = call-poly <vilib>:"CTRE_Phoenix_MotorController_Get_Enhanced.vi"("PhoenixMotorControlDevRef"=w2) -> ("Quadrature Position"=w3:i32)  [unwired: 11 in, 3 out]
  n24 = disable-structure shown="Disabled" {
    disable-tunnel: [w116 _] -> w29
    frame Disabled {
      n25 = call <vilib>:"WPI_GyroRefNum Registry Get.vi"("refnum name"="Gyro") -> ("GyroDevRef"=w116:T20)  [unwired: 9 in, 1 out]
    }
    frame Enabled {
    }
  }
  n26 = global write "Robot Global Data.vi" "HAB Bk Spd Encoder Start Value"(w3) -> ()
  n27 = Bundle("DriveJoystickDevRef"="DriveJoystickDevRef", "AuxJoystickDevRef"="AuxJoystickDevRef", "Drive Axes"=w107, "Drive Buttons"=w106, "Drive POVs"=w105, "Aux Axes"=w104, "Aux Buttons"=w103, "Aux POVs"=w102, "Robot Mode"=w101, "Drive Motors"="Drive Motors", "Drive Joystick Indexes"=w97, "Drive Button Indexes"=w95, "Joystick VS Vision Latch"=w94, "Vision States"=w93, "limelight"=w92, "Vision Track Mode Override"=w91, "T = Motion Profile, F = Percent Output"=w28) -> (w111:T23)  [unwired: 1 in]
  n28 = Bundle By Name(cluster=w111, "Drive Motors"=w99, "DriveJoystickDevRef"=w110, "AuxJoystickDevRef"=w109) -> (w108:T23)
  n29 = global write "Robot Global Data.vi" "Hatch Encoder Start Value"(w62) -> ()
  n30 = Bundle("TopRetainerSwitchDevRef"="TopRetainerSwitchDevRef", "BottomRetainerSwitchDevRef"="BottomRetainerSwitchDevRef", "HatchRetainerMotorDevRef"="HatchRetainerMotorDevRef", "LifterSolenoidDevRef"="LifterSolenoidDevRef", "DriveJoystickDevRef"="DriveJoystickDevRef", "KickerSolenoidDevRef"="KickerSolenoidDevRef", "RetainerSolenoidDevRef"="RetainerSolenoidDevRef", "AuxJoystickDevRef"="AuxJoystickDevRef", "HatchCollectorMotorDevRef"="HatchCollectorMotorDevRef", "Drive Axes"=w77, "Drive Buttons"=w76, "Drive POVs"=w75, "Aux Axes"=w74, "Aux Buttons"=w73, "Aux POVs"=w72, "Robot Mode"=w71, "Aux Joystick Indexes"=w67, "Aux Button Indexes"=w66, "Hatch Retainer Move Up/Down"=w65, "Hatch Collector Actual Angle"=w64, "Hatch Collector Wanted Angle"=w30, "Hatch Retainer States"=w18) -> (w88:T24)  [unwired: 1 in]
  n31 = Bundle By Name(cluster=w88, "TopRetainerSwitchDevRef"=w19, "BottomRetainerSwitchDevRef"=w20, "HatchRetainerMotorDevRef"=w25, "HatchCollectorMotorDevRef"=w63, "DriveJoystickDevRef"=w68, "AuxJoystickDevRef"=w82, "KickerSolenoidDevRef"=w85, "RetainerSolenoidDevRef"=w84, "LifterSolenoidDevRef"=w60) -> (w78:T24)
  n32 = Bundle("BkSpdAdjusterMotorDevRef"="BkSpdAdjusterMotorDevRef", "HABAssisterSolenoidDevRef"="HABAssisterSolenoidDevRef", "Back HAB 3 Limit Switch"="Back HAB 3 Limit Switch", "Front HAB 3 Limit Switch"="Front HAB 3 Limit Switch", "HAB3DriveModuleMotorDevRef"="HAB3DriveModuleMotorDevRef", "DriveJoystickDevRef"="DriveJoystickDevRef", "AuxJoystickDevRef"="AuxJoystickDevRef", "HAB3FrontSolenoidDevRef"="HAB3FrontSolenoidDevRef", "HAB3BackSolenoidDevRef"="HAB3BackSolenoidDevRef", "Drive Axes"=w41, "Drive Buttons"=w40, "Drive POVs"=w39, "Aux Axes"=w38, "Aux Buttons"=w37, "Aux POVs"=w36, "Robot Mode"=w35, "Aux Joystick Indexes"=w34, "Aux Button Indexes"=w33, "Front Cylinders Latch"=w32, "Back Cylinders Latch"=w31, "Yaw"=w8, "Pitch"=w7, "Roll"=w6, "HAB Bk Spd Motor States"=w1) -> (w48:T25)  [unwired: 1 in]
  n33 = Bundle By Name(cluster=w48, "BkSpdAdjusterMotorDevRef"=w2, "HABAssisterSolenoidDevRef"=w9, "Front HAB 3 Limit Switch"=w13, "Back HAB 3 Limit Switch"=w12, "HAB3DriveModuleMotorDevRef"=w43, "DriveJoystickDevRef"=w44, "AuxJoystickDevRef"=w45, "HAB3FrontSolenoidDevRef"=w46, "HAB3BackSolenoidDevRef"=w47) -> (w42:T25)
  n34 = while {
    shift-right: [w142] -> _
    shift-left: w78 -> [w183]
    stop <- FALSE stop-if-true
    # "it's back-\nwards"
    # "this chunk of code \ncontrols the wanted\nangle of the collector\nusing a joystick and\n2 angle presets"
    # "use this to scale the rate at which the\nwanted angle changes based on the joystick"
    # "we use this to set the\n\"0\" of the encoder to be \nwherever it is when the code\nis run (or the robot is turned\non in the case of \nhard-deployed code)"
    # "this chunk of code \nconverts the encoder\n values into angles"
    # "*** might want to make it so it stays extended\nfor set amount of time instead of however\nlong the driver is holding the button ***"
    n35 = Unbundle By Name(w183) -> ("DriveJoystickDevRef"=w194:T9)
    n36 = Unbundle By Name(w183) -> ("AuxJoystickDevRef"=w193:T9)
    n37 = Unbundle By Name(w183) -> ("Robot Mode"=w192:T16)
    n38 = Wait (ms)(milliseconds to wait=u32 50) -> ()  [unwired: 1 out]
    n39 = call <vilib>:"WPI_JoystickGetValues.vi"("JoystickDevRef"=w193) -> ("Buttons"=w185:bool[], "Axes"=w186:dbl[], "JoystickDevRef"=w187:T9, "POVs"=w184:i16[])  [unwired: 6 in, 1 out]
    n40 = call <vilib>:"WPI_JoystickGetValues.vi"("JoystickDevRef"=w194) -> ("Buttons"=w189:bool[], "Axes"=w191:dbl[], "JoystickDevRef"=w190:T9, "POVs"=w188:i16[])  [unwired: 6 in, 1 out]
    n41 = case shown="\"Teleop Enabled\"" w192 {
      tunnel: w183 -> [w296 w306 w307 w308 w318 w319 w320 w330 w331]
      tunnel: [w296 w297 w307 w309 w318 w319 w320 w321 w331] -> w154
      tunnel: w191 -> [_ w305 _ w316 _ _ _ w328 _]
      tunnel: w190 -> [_ w304 _ w317 _ _ _ w329 _]
      tunnel: w189 -> [_ w303 _ w315 _ _ _ w327 _]
      tunnel: w188 -> [_ w302 _ w314 _ _ _ w326 _]
      tunnel: w187 -> [_ w301 _ w313 _ _ _ w325 _]
      tunnel: w186 -> [_ w300 _ w312 _ _ _ w324 _]
      tunnel: w185 -> [_ w299 _ w311 _ _ _ w323 _]
      tunnel: w184 -> [_ w298 _ w310 _ _ _ w322 _]
      frame "Autonomous Disabled", Default {
      }
      frame "Autonomous Enabled" {
        n42 = Bundle By Name(cluster=w306, "DriveJoystickDevRef"=w304, "Drive Axes"=w305, "Drive Buttons"=w303, "Drive POVs"=w302, "AuxJoystickDevRef"=w301, "Aux Axes"=w300, "Aux Buttons"=w299, "Aux POVs"=w298) -> (w297:T24)
      }
      frame "Teleop Disabled" {
      }
      frame "Teleop Enabled" {
        n43 = Bundle By Name(cluster=w308, "DriveJoystickDevRef"=w317, "Drive Axes"=w316, "Drive Buttons"=w315, "Drive POVs"=w314, "AuxJoystickDevRef"=w313, "Aux Axes"=w312, "Aux Buttons"=w311, "Aux POVs"=w310) -> (w309:T24)
      }
      frame "Disconnected" {
      }
      frame "Finish" {
      }
      frame "Test Disabled" {
      }
      frame "Test Enabled" {
        n44 = Bundle By Name(cluster=w330, "DriveJoystickDevRef"=w329, "Drive Axes"=w328, "Drive Buttons"=w327, "Drive POVs"=w326, "AuxJoystickDevRef"=w325, "Aux Axes"=w324, "Aux Buttons"=w323, "Aux POVs"=w322) -> (w321:T24)
      }
      frame "Emergency Stopped" {
      }
    }
    n45 = Unbundle By Name(w154) -> ("Aux Button Indexes.Y Button"=w152:i32)
    n46 = Unbundle By Name(w154) -> ("Aux Button Indexes.X Button"=w151:i32)
    n47 = Unbundle By Name(w154) -> ("Aux Axes"=w162:dbl[])
    n48 = Unbundle By Name(w154) -> ("Aux Buttons"=w153:bool[])
    n49 = Unbundle By Name(w154) -> ("Aux Button Indexes.A Button"=w175:i32)
    n50 = Unbundle By Name(w154) -> ("Aux Buttons"=w174:bool[])
    n51 = Unbundle By Name(w154) -> ("Hatch Collector Wanted Angle"=w159:dbl)
    n52 = Unbundle By Name(w154) -> ("Aux Joystick Indexes.Left Y"=w161:i32)
    n53 = Unbundle By Name(w154) -> ("Hatch Retainer Move Up/Down"=w171:bool)
    n54 = Unbundle By Name(w154) -> ("HatchCollectorMotorDevRef"=w168:T1)
    n55 = global read "Robot Global Data.vi" "Hatch Encoder Start Value"() -> (w163:dbl)
    n56 = global read "Robot Global Data.vi" "Robot Mode"() -> (w182:T16)
    n57 = global read "Robot Global Data.vi" "Which Robot?"() -> (w130:T28)
    n58 = Bundle By Name(cluster=w154, "Robot Mode"=w182) -> (w173:T24)
    n59 = call-poly <vilib>:"CTRE_Phoenix_MotorController_Get_Enhanced.vi"("PhoenixMotorControlDevRef"=w168) -> ("Quadrature Position"=w166:i32)  [unwired: 11 in, 3 out]
    n60 = Index Array(array=w162, index=w161) -> (element=w145:dbl)
    n61 = Index Array(array=w174, index=w175) -> (element=w172:bool)
    n62 = Index Array(array=w153, index #1=w152, index #2=w151) -> (element #1=w148:bool, element #2=w149:bool)
    n63 = call "Deadband.vi"("Input"=w145) -> ("Output"=w144:dbl)  [unwired: 10 in]
    n64 = disable-structure shown="Enabled" {
      disable-tunnel: w172 -> [w212 w216]
      disable-tunnel: w171 -> [w209 _]
      disable-tunnel: [w208 w215] -> w170
      frame Disabled {
        n65 = feedback #1() -> (w213:bool)  [unwired: 1 in]
        n66 = feedback-in #1(w212) -> ()
        n67 = Greater?(x=w212, y=w213) -> (0:w211:bool)
        n68 = Not(x=w209) -> (.not. x?=w210:bool)
        n69 = Select(t=w210, s=w211, f=w209) -> (s? t:f=w208:bool)
      }
      frame Enabled {
        n70 = feedback #2() -> (w214:bool)  [unwired: 1 in]
        n71 = feedback-in #2(w216) -> ()
        n72 = Greater?(x=w216, y=w214) -> (0:w215:bool)
      }
    }
    n73 = case shown="\"Competition Bot\", Default" w130 {
      tunnel: [w271 w280 w289] -> w167
      tunnel: w166 -> [w269 w279 w288]
      tunnel: w163 -> [w270 w278 w287]
      frame "Competition Bot", Default {
        # "range of \ndegrees"
        # "enc. val at\n\"max out\"\ndeg IRL"
        # "enc. val at\n\"max in\"\ndeg IRL"
        n74 = Subtract(x=w269, y=w270) -> (x-y=w272:dbl)
        n75 = Subtract(x=1047.0, y=46.0) -> (x-y=w276:dbl)
        n76 = Divide(x=97.0, y=w276) -> (x/y=w274:dbl)
        n77 = Multiply(x=w274, y=w272) -> (x*y=w271:dbl)
      }
      frame "Practice Bot" {
        # "range of \ndegrees"
        # "enc. val at\n\"max out\"\ndeg IRL"
        # "enc. val at\n\"max in\"\ndeg IRL"
        n78 = Subtract(x=w279, y=w278) -> (x-y=w281:dbl)
        n79 = Subtract(x=1050.0, y=34.0) -> (x-y=w285:dbl)
        n80 = Divide(x=90.0, y=w285) -> (x/y=w283:dbl)
        n81 = Multiply(x=w283, y=w281) -> (x*y=w280:dbl)
      }
      frame "Code Bot" {
        # "range of \ndegrees"
        # "enc. val at\n\"max out\"\ndeg IRL"
        # "enc. val at\n\"max in\"\ndeg IRL"
        n82 = Subtract(x=w288, y=w287) -> (x-y=w290:dbl)
        n83 = Subtract(x=1050.0, y=34.0) -> (x-y=w294:dbl)
        n84 = Divide(x=90.0, y=w294) -> (x/y=w292:dbl)
        n85 = Multiply(x=w292, y=w290) -> (x*y=w289:dbl)
      }
    }
    n86 = Negate(x=w144) -> (-x=w134:dbl)
    n87 = Add(x=w159, y=w134) -> (x+y=w158:dbl)
    n88 = Or(x=w148, y=w149) -> (x .or. y?=w150:bool)
    n89 = Multiply(x=1.0, y=w158) -> (x*y=w155:dbl)
    n90 = case shown="True" w150 {
      tunnel: [w264 w265] -> w156
      tunnel: w155 -> [w264 _]
      tunnel: w148 -> [_ w266]
      frame False {
        # "neither \npreset,\nJS controls\nwanted angle"
      }
      frame True {
        n91 = case shown="True" w266 {
          tunnel: [80.0 7.0] -> w265
          frame False {
            # "preset \nfor \nhovering\nto use \ndustpan"
          }
          frame True {
            # "preset\nfor \nvertical"
          }
        }
      }
    }
    n92 = global read "Robot Global Data.vi" "Which Robot?"() -> (w129:T28)
    n93 = case shown="\"Competition Bot\", Default" w129 {
      tunnel: [97.0 99.0 90.0] -> w128
      frame "Competition Bot", Default {
        # "max deg"
      }
      frame "Practice Bot" {
        # "max deg"
      }
      frame "Code Bot" {
        # "max deg"
      }
    }
    n94 = In Range and Coerce(upper limit=w128, x=w156, lower limit=0.0) -> (coerced(x)=w147:dbl)  [unwired: 1 out]
    n95 = Bundle By Name(cluster=w173, "Hatch Retainer Move Up/Down"=w170) -> (w169:T24)
    n96 = Bundle By Name(cluster=w169, "Hatch Collector Actual Angle"=w167) -> (w160:T24)
    n97 = Bundle By Name(cluster=w160, "Hatch Collector Wanted Angle"=w147) -> (w118:T24)
    n98 = disable-structure shown="Disabled" {
      disable-tunnel: w118 -> [w250 _]
      frame Disabled {
        n99 = Unbundle By Name(w250) -> ("RetainerSolenoidDevRef"=w255:T6)
        n100 = Unbundle By Name(w250) -> ("Hatch Retainer Move Up/Down"=w251:bool)
        n101 = Select(t=WPI_SolenoidValue."On" ("Value"), s=w251, f=WPI_SolenoidValue."Off" ("Value")) -> (s? t:f=w254:T26)
        n102 = call-poly <vilib>:"WPI_SolenoidSet.vi"("Value"=w254, "SolenoidDevRef"=w255) -> ()  [unwired: 8 in, 2 out]
      }
      frame Enabled {
      }
    }
    n103 = Unbundle By Name(w118) -> ("KickerSolenoidDevRef"=w181:T6)
    n104 = Unbundle By Name(w118) -> ("Aux Button Indexes.RB Button"=w179:i32)
    n105 = disable-structure shown="Disabled" {
      disable-tunnel: w118 -> [w256 _]
      frame Disabled {
        n106 = Unbundle By Name(w256) -> ("Aux Button Indexes.B Button"=w263:i32)
        n107 = Unbundle By Name(w256) -> ("LifterSolenoidDevRef"=w257:T6)
        n108 = Unbundle By Name(w256) -> ("Aux Buttons"=w262:bool[])
        n109 = Index Array(array=w262, index=w263) -> (element=w259:bool)
        n110 = Select(t=WPI_SolenoidValue."On" ("Value"), s=w259, f=WPI_SolenoidValue."Off" ("Value")) -> (s? t:f=w258:T26)
        n111 = call-poly <vilib>:"WPI_SolenoidSet.vi"("Value"=w258, "SolenoidDevRef"=w257) -> ()  [unwired: 8 in, 2 out]
      }
      frame Enabled {
      }
    }
    n112 = Unbundle By Name(w118) -> ("Aux Buttons"=w180:bool[])
    n113 = global read "Robot Global Data.vi" "Kick Hatch in Auto"() -> (w125:bool)
    n114 = Index Array(array=w180, index=w179) -> (element=w127:bool)
    n115 = Or(x=w127, y=w125) -> (x .or. y?=w126:bool)
    n116 = Select(t=WPI_SolenoidValue."On" ("Value"), s=w126, f=WPI_SolenoidValue."Off" ("Value")) -> (s? t:f=w176:T26)
    n117 = call-poly <vilib>:"WPI_SolenoidSet.vi"("Value"=w176, "SolenoidDevRef"=w181) -> ()  [unwired: 8 in, 2 out]
    n118 = global read "Robot Global Data.vi" "Which Robot?"() -> (w133:T28)
    n119 = Unbundle By Name(w118) -> ("BottomRetainerSwitchDevRef"=w137:T8)
    n120 = global read "Robot Global Data.vi" "Which Robot?"() -> (w132:T28)
    n121 = Unbundle By Name(w118) -> ("Hatch Collector Wanted Angle"=w121:dbl)
    n122 = Unbundle By Name(w118) -> ("Hatch Collector Actual Angle"=w120:dbl)
    n123 = Unbundle By Name(w118) -> ("Hatch Retainer States"=w143:T13)
    n124 = Unbundle By Name(w118) -> ("HatchRetainerMotorDevRef"=w135:T1)
    n125 = Unbundle By Name(w118) -> ("Hatch Retainer Move Up/Down"=w140:bool)
    n126 = Unbundle By Name(w118) -> ("TopRetainerSwitchDevRef"=w139:T8)
    n127 = case shown="\"Competition Bot\", Default" w132 {
      tunnel: [w203 T27 {"proportional gain (Kc)"=0.0, "integral time (Ti, min)"=0.0, "derivative time (Td, min)"=0.0} ("PID gains") T27 {"proportional gain (Kc)"=0.004, "integral time (Ti, min)"=0.0, "derivative time (Td, min)"=0.0} ("PID gains")] -> w131
      frame "Competition Bot", Default {
        # "9.7% motor speed seems\nto be minimum to move"
        n128 = disable-structure shown="Enabled" {
          disable-tunnel: [T27 {"proportional gain (Kc)"=0.03, "integral time (Ti, min)"=0.003, "derivative time (Td, min)"=0.0} ("PID gains") T27 {"proportional gain (Kc)"=0.035, "integral time (Ti, min)"=0.0, "derivative time (Td, min)"=0.0} ("PID gains")] -> w203
          frame Disabled {
          }
          frame Enabled {
          }
        }
      }
      frame "Practice Bot" {
      }
      frame "Code Bot" {
        # "p = 0.008 is WAY too fast"
        # "for code bot:\nwe ended with p = 0.004,\nbut the motor has to turn\nso slowly on the code bot\nthat no PID values would\nreally work well"
      }
    }
    n129 = case shown="\"Competition Bot\", Default" w133 {
      tunnel: [cluster{"output high":dbl, "output low":dbl} {"output high"=0.2, "output low"=-0.4} ("output range") cluster{"output high":dbl, "output low":dbl} {"output high"=0.15, "output low"=-0.15} ("output range") cluster{"output high":dbl, "output low":dbl} {"output high"=0.15, "output low"=-0.15} ("output range")] -> w119
      frame "Competition Bot", Default {
      }
      frame "Practice Bot" {
      }
      frame "Code Bot" {
      }
    }
    n130 = call <vilib>:"WPI_DigitalInputGetValue.vi"("DigitalInputDevRef"=w139) -> ("Value"=w138:bool)  [unwired: 8 in, 2 out]
    n131 = call <vilib>:"WPI_DigitalInputGetValue.vi"("DigitalInputDevRef"=w137) -> ("Value"=w136:bool)  [unwired: 8 in, 2 out]
    n132 = call-poly <vilib>:"PID.vi"("output range"=w119, "PID gains"=w131, "process variable"=w120, "setpoint"=w121) -> ("output"=w164:dbl)  [unwired: 6 in, 1 out]
    n133 = Not(x=w136) -> (.not. x?=w123:bool)
    n134 = Not(x=w138) -> (.not. x?=w124:bool)
    n135 = Unbundle By Name(w118) -> ("HatchCollectorMotorDevRef"=w165:T1)
    n136 = case shown="\"Going Down\"" w143 {
      tunnel: [w220 w225 w239 w244] -> w141
      tunnel: w140 -> [w223 _ w240 _]
      tunnel: w124 -> [_ w227 _ _]
      tunnel: w123 -> [_ _ _ w243]
      tunnel: w135 -> [w217 w226 w235 w242]
      tunnel: 0.2 ("Output") -> [_ w224 _ w241]
      frame "Fully Down", Default {
        w219 = T29 0 items=["PercentOutput"=0, "Position"=1, "Velocity"=2, "Current"=3, "Follower"=5, "MotionProfile"=6, "MotionMagic"=7, "MotionProfileArc"=10, "Disabled"=15] ("Control Mode")
        n137 = Select(t=Hatch_Retainer_States."Going Up" ("Hatch Retainer States"), s=w223, f=Hatch_Retainer_States."Fully Down" ("Hatch Retainer States")) -> (s? t:f=w220:T13)
        n138 = call <vilib>:"CTRE_Phoenix_MotorControl_Set.vi"("Output"=0.0, "Control Mode"=w219, "PhoenixMotorControlDevRef"=w217) -> ()  [unwired: 7 in, 2 out]
      }
      frame "Going Up" {
        n139 = case shown="True" w227 {
          tunnel: w226 -> [w232 _]
          tunnel: [Hatch_Retainer_States."Going Up" ("Hatch Retainer States") Hatch_Retainer_States."Fully Up" ("Hatch Retainer States")] -> w225
          tunnel: w224 -> [w229 _]
          frame False {
            w230 = T29 0 items=["PercentOutput"=0, "Position"=1, "Velocity"=2, "Current"=3, "Follower"=5, "MotionProfile"=6, "MotionMagic"=7, "MotionProfileArc"=10, "Disabled"=15] ("Control Mode")
            n140 = Negate(x=w229) -> (-x=w228:dbl)
            n141 = call <vilib>:"CTRE_Phoenix_MotorControl_Set.vi"("Output"=w228, "Control Mode"=w230, "PhoenixMotorControlDevRef"=w232) -> ()  [unwired: 7 in, 2 out]
          }
          frame True {
          }
        }
      }
      frame "Fully Up" {
        w236 = T29 0 items=["PercentOutput"=0, "Position"=1, "Velocity"=2, "Current"=3, "Follower"=5, "MotionProfile"=6, "MotionMagic"=7, "MotionProfileArc"=10, "Disabled"=15] ("Control Mode")
        n142 = call <vilib>:"CTRE_Phoenix_MotorControl_Set.vi"("Output"=0.0, "Control Mode"=w236, "PhoenixMotorControlDevRef"=w235) -> ()  [unwired: 7 in, 2 out]
        n143 = Select(t=Hatch_Retainer_States."Going Down" ("Hatch Retainer States"), s=w240, f=Hatch_Retainer_States."Fully Up" ("Hatch Retainer States")) -> (s? t:f=w239:T13)
      }
      frame "Going Down" {
        n144 = case shown="False" w243 {
          tunnel: [Hatch_Retainer_States."Going Down" ("Hatch Retainer States") Hatch_Retainer_States."Fully Down" ("Hatch Retainer States")] -> w244
          tunnel: w242 -> [w247 _]
          tunnel: w241 -> [w245 _]
          frame False {
            w246 = T29 0 items=["PercentOutput"=0, "Position"=1, "Velocity"=2, "Current"=3, "Follower"=5, "MotionProfile"=6, "MotionMagic"=7, "MotionProfileArc"=10, "Disabled"=15] ("Control Mode")
            n145 = call <vilib>:"CTRE_Phoenix_MotorControl_Set.vi"("Output"=w245, "Control Mode"=w246, "PhoenixMotorControlDevRef"=w247) -> ()  [unwired: 7 in, 2 out]
          }
          frame True {
          }
        }
      }
    }
    n146 = call <vilib>:"WPI_MotorControlSetOutput.vi"("Output"=w164, "MotorControlDevRef"=w165) -> ()  [unwired: 7 in, 3 out]
    n147 = Bundle By Name(cluster=w118, "Hatch Retainer States"=w141) -> (w142:T24)
  }
  n148 = while {
    shift-right: [w332] -> _
    shift-left: w42 -> [w380]
    stop <- FALSE stop-if-true
    w349 = T29 2 items=["PercentOutput"=0, "Position"=1, "Velocity"=2, "Current"=3, "Follower"=5, "MotionProfile"=6, "MotionMagic"=7, "MotionProfileArc"=10, "Disabled"=15] ("Control Mode")
    # "would slow down if pos. pitch, \nwhich is opposite of what we want"
    # "base spd +- PID adjustments"
    # "they're inverted\nfor some \nreason?"
    n149 = Unbundle By Name(w380) -> ("DriveJoystickDevRef"=w391:T9)
    n150 = Unbundle By Name(w380) -> ("AuxJoystickDevRef"=w390:T9)
    n151 = Unbundle By Name(w380) -> ("Robot Mode"=w389:T16)
    n152 = call <vilib>:"WPI_JoystickGetValues.vi"("JoystickDevRef"=w390) -> ("Buttons"=w382:bool[], "Axes"=w383:dbl[], "JoystickDevRef"=w384:T9, "POVs"=w381:i16[])  [unwired: 6 in, 1 out]
    n153 = call <vilib>:"WPI_JoystickGetValues.vi"("JoystickDevRef"=w391) -> ("Buttons"=w386:bool[], "Axes"=w388:dbl[], "JoystickDevRef"=w387:T9, "POVs"=w385:i16[])  [unwired: 6 in, 1 out]
    n154 = Wait (ms)(milliseconds to wait=50) -> ()  [unwired: 1 out]
    n155 = case shown="\"Teleop Enabled\"" w389 {
      tunnel: w380 -> [w517 w527 w528 w529 w539 w540 w541 w551 w552]
      tunnel: [w517 w518 w528 w530 w539 w540 w541 w542 w552] -> w358
      tunnel: w388 -> [_ w526 _ w537 _ _ _ w549 _]
      tunnel: w387 -> [_ w525 _ w538 _ _ _ w550 _]
      tunnel: w386 -> [_ w524 _ w536 _ _ _ w548 _]
      tunnel: w385 -> [_ w523 _ w535 _ _ _ w547 _]
      tunnel: w384 -> [_ w522 _ w534 _ _ _ w546 _]
      tunnel: w383 -> [_ w521 _ w533 _ _ _ w545 _]
      tunnel: w382 -> [_ w520 _ w532 _ _ _ w544 _]
      tunnel: w381 -> [_ w519 _ w531 _ _ _ w543 _]
      frame "Autonomous Disabled", Default {
      }
      frame "Autonomous Enabled" {
        n156 = Bundle By Name(cluster=w527, "DriveJoystickDevRef"=w525, "Drive Axes"=w526, "Drive Buttons"=w524, "Drive POVs"=w523, "AuxJoystickDevRef"=w522, "Aux Axes"=w521, "Aux Buttons"=w520, "Aux POVs"=w519) -> (w518:T25)
      }
      frame "Teleop Disabled" {
      }
      frame "Teleop Enabled" {
        n157 = Bundle By Name(cluster=w529, "DriveJoystickDevRef"=w538, "Drive Axes"=w537, "Drive Buttons"=w536, "Drive POVs"=w535, "AuxJoystickDevRef"=w534, "Aux Axes"=w533, "Aux Buttons"=w532, "Aux POVs"=w531) -> (w530:T25)
      }
      frame "Disconnected" {
      }
      frame "Finish" {
      }
      frame "Test Disabled" {
      }
      frame "Test Enabled" {
        n158 = Bundle By Name(cluster=w551, "DriveJoystickDevRef"=w550, "Drive Axes"=w549, "Drive Buttons"=w548, "Drive POVs"=w547, "AuxJoystickDevRef"=w546, "Aux Axes"=w545, "Aux Buttons"=w544, "Aux POVs"=w543) -> (w542:T25)
      }
      frame "Emergency Stopped" {
      }
    }
    n159 = global read "Robot Global Data.vi" "Robot Mode"() -> (w362:T16)
    n160 = Bundle By Name(cluster=w358, "Robot Mode"=w362) -> (w361:T25)
    n161 = disable-structure shown="Enabled" {
      disable-tunnel: w361 -> [w431 w475]
      disable-tunnel: w358 -> [w430 w477]
      disable-tunnel: [_ w462] -> w333
      frame Disabled {
        # "disabled because the RT code would override the instructions of the LT and LB code using separate bundle by names"
        # "controls both \ncylinders together"
        # "controls back cylinders only"
        # "controls front cylinders only"
        n162 = Unbundle By Name(w430) -> ("Aux Button Indexes.RT Button"=w444:i32)
        n163 = Unbundle By Name(w430) -> ("Aux Buttons"=w443:bool[])
        n164 = Unbundle By Name(w430) -> ("Aux Button Indexes.LT Button"=w446:i32)
        n165 = Unbundle By Name(w430) -> ("Front Cylinders Latch"=w439:bool)
        n166 = Unbundle By Name(w430) -> ("Aux Button Indexes.LB Button"=w461:i32)
        n167 = Unbundle By Name(w430) -> ("Aux Buttons"=w447:bool[])
        n168 = Unbundle By Name(w430) -> ("Back Cylinders Latch"=w436:bool)
        n169 = Unbundle By Name(w430) -> ("Aux Buttons"=w460:bool[])
        n170 = Unbundle By Name(w430) -> ("Back Cylinders Latch"=w452:bool)
        n171 = Unbundle By Name(w430) -> ("Front Cylinders Latch"=w455:bool)
        n172 = Index Array(array=w443, index=w444) -> (element=w441:bool)
        n173 = Index Array(array=w447, index=w446) -> (element=w449:bool)
        n174 = Index Array(array=w460, index=w461) -> (element=w458:bool)
        n175 = feedback #3() -> (w442:bool)  [unwired: 1 in]
        n176 = feedback-in #3(w441) -> ()
        n177 = feedback #4() -> (w448:bool)  [unwired: 1 in]
        n178 = feedback-in #4(w449) -> ()
        n179 = feedback #5() -> (w459:bool)  [unwired: 1 in]
        n180 = feedback-in #5(w458) -> ()
        n181 = Greater?(x=w441, y=w442) -> (0:w435:bool)
        n182 = Greater?(x=w449, y=w448) -> (0:w450:bool)
        n183 = Greater?(x=w458, y=w459) -> (0:w457:bool)
        n184 = Not(x=w436) -> (.not. x?=w437:bool)
        n185 = Not(x=w439) -> (.not. x?=w440:bool)
        n186 = Not(x=w452) -> (.not. x?=w451:bool)
        n187 = Not(x=w455) -> (.not. x?=w456:bool)
        n188 = Select(t=w437, s=w435, f=w436) -> (s? t:f=w434:bool)
        n189 = Select(t=w440, s=w435, f=w439) -> (s? t:f=w438:bool)
        n190 = Select(t=w451, s=w450, f=w452) -> (s? t:f=w453:bool)
        n191 = Select(t=w456, s=w457, f=w455) -> (s? t:f=w454:bool)
        n192 = Bundle By Name(cluster=w431, "Front Cylinders Latch"=w454) -> (w445:T25)
        n193 = Bundle By Name(cluster=w445, "Back Cylinders Latch"=w453) -> (w433:T25)
        n194 = Bundle By Name(cluster=w433, "Front Cylinders Latch"=w438) -> (w432:T25)
        n195 = Bundle By Name(cluster=w432, "Back Cylinders Latch"=w434) -> (w429:T25)
      }
      frame Enabled {
        # "controls both \ncylinders together"
        # "controls back cylinders only"
        # "controls front cylinders only"
        n196 = Unbundle By Name(w477) -> ("Aux Button Indexes.RT Button"=w481:i32)
        n197 = Unbundle By Name(w477) -> ("Aux Buttons"=w480:bool[])
        n198 = Unbundle By Name(w477) -> ("Aux Button Indexes.LT Button"=w482:i32)
        n199 = Unbundle By Name(w477) -> ("Aux Button Indexes.LB Button"=w489:i32)
        n200 = Unbundle By Name(w477) -> ("Aux Buttons"=w483:bool[])
        n201 = Unbundle By Name(w477) -> ("Aux Buttons"=w488:bool[])
        n202 = Unbundle By Name(w477) -> ("Front Cylinders Latch"=w468:bool)
        n203 = Unbundle By Name(w477) -> ("Back Cylinders Latch"=w465:bool)
        n204 = Index Array(array=w480, index=w481) -> (element=w478:bool)
        n205 = Index Array(array=w483, index=w482) -> (element=w485:bool)
        n206 = Index Array(array=w488, index=w489) -> (element=w486:bool)
        n207 = feedback #6() -> (w479:bool)  [unwired: 1 in]
        n208 = feedback-in #6(w478) -> ()
        n209 = feedback #7() -> (w484:bool)  [unwired: 1 in]
        n210 = feedback-in #7(w485) -> ()
        n211 = feedback #8() -> (w487:bool)  [unwired: 1 in]
        n212 = feedback-in #8(w486) -> ()
        n213 = Greater?(x=w478, y=w479) -> (0:w472:bool)
        n214 = Greater?(x=w485, y=w484) -> (0:w473:bool)
        n215 = Greater?(x=w486, y=w487) -> (0:w474:bool)
        n216 = Or(x=w474, y=w472) -> (x .or. y?=w471:bool)
        n217 = Or(x=w473, y=w472) -> (x .or. y?=w466:bool)
        n218 = Not(x=w468) -> (.not. x?=w469:bool)
        n219 = Not(x=w465) -> (.not. x?=w467:bool)
        n220 = Select(t=w469, s=w471, f=w468) -> (s? t:f=w470:bool)
        n221 = Select(t=w467, s=w466, f=w465) -> (s? t:f=w464:bool)
        n222 = Bundle By Name(cluster=w475, "Front Cylinders Latch"=w470) -> (w476:T25)
        n223 = Bundle By Name(cluster=w476, "Back Cylinders Latch"=w464) -> (w463:T25)
        n224 = disable-structure shown="Disabled" {
          disable-tunnel: w463 -> [w494 w496]
          disable-tunnel: [w493 w496] -> w462
          frame Disabled {
            # "yaw is the angle of our robot\npitch is the angle of elevation of our robot\nroll is how much the robot is rotated about its center"
            n225 = call <vilib>:"Get_YPRHfH.vi"() -> ("YRPHfH"=w495:T30)  [unwired: 11 in]
            n226 = Unbundle By Name(w495) -> ("Yaw"=w492:dbl)
            n227 = Unbundle By Name(w495) -> ("Pitch"=w491:dbl)
            n228 = Unbundle By Name(w495) -> ("Roll"=w490:dbl)
            n229 = global write "Robot Global Data.vi" "Yaw (clockwise/counter-clockwise)"(w492) -> ()
            n230 = global write "Robot Global Data.vi" "Roll (forward/backward tipping)"(w490) -> ()
            n231 = global write "Robot Global Data.vi" "Pitch (left/right tipping)"(w491) -> ()
            n232 = Bundle By Name(cluster=w494, "Yaw"=w492, "Pitch"=w491, "Roll"=w490) -> (w493:T25)
          }
          frame Enabled {
          }
        }
      }
    }
    n233 = Unbundle By Name(w333) -> ("Pitch"=w355:dbl)
    n234 = Unbundle By Name(w333) -> ("HAB3FrontSolenoidDevRef"=w379:T6)
    n235 = global read "Robot Global Data.vi" "Which Robot?"() -> (w353:T28)
    n236 = Unbundle By Name(w333) -> ("HABAssisterSolenoidDevRef"=w357:T6)
    n237 = Unbundle By Name(w333) -> ("Front Cylinders Latch"=w376:bool)
    n238 = Unbundle By Name(w333) -> ("HAB3BackSolenoidDevRef"=w372:T6)
    n239 = Unbundle By Name(w333) -> ("BkSpdAdjusterMotorDevRef"=w346:T1)
    n240 = Unbundle By Name(w333) -> ("HAB Bk Spd Motor States"=w343:T12)
    n241 = Unbundle By Name(w333) -> ("Back Cylinders Latch"=w342:bool)
    n242 = global read "Robot Global Data.vi" "Which Robot?"() -> (w351:T28)
    n243 = case shown="\"Competition Bot\", Default" w351 {
      tunnel: [cluster{"output high":dbl, "output low":dbl} {"output high"=0.2, "output low"=-0.4} ("output range") cluster{"output high":dbl, "output low":dbl} {"output high"=0.15, "output low"=-0.15} ("output range") cluster{"output high":dbl, "output low":dbl} {"output high"=0.15, "output low"=-0.15} ("output range")] -> w350
      frame "Competition Bot", Default {
      }
      frame "Practice Bot" {
      }
      frame "Code Bot" {
      }
    }
    n244 = case shown="\"Code Bot\"" w353 {
      tunnel: [T27 {"proportional gain (Kc)"=0.0, "integral time (Ti, min)"=0.0, "derivative time (Td, min)"=0.0} ("PID gains") T27 {"proportional gain (Kc)"=0.0, "integral time (Ti, min)"=0.0, "derivative time (Td, min)"=0.0} ("PID gains") T27 {"proportional gain (Kc)"=0.0, "integral time (Ti, min)"=0.0, "derivative time (Td, min)"=0.0} ("PID gains")] -> w352
      tunnel: [w423 w425 w427] -> w340
      frame "Competition Bot", Default {
        w423 = 0.0  # Enc. Val at Fully Down
      }
      frame "Practice Bot" {
        w425 = 0.0  # Enc. Val at Fully Down
      }
      frame "Code Bot" {
        w427 = 0.0  # Enc. Val at Fully Down
      }
    }
    n245 = call-poly <vilib>:"PID.vi"("output range"=w350, "PID gains"=w352, "process variable"=w355, "setpoint"=0.0) -> ("output"=w348:dbl)  [unwired: 6 in, 1 out]
    n246 = global read "Robot Global Data.vi" "HAB Bk Spd Encoder Start Value"() -> (w344:dbl)
    n247 = Negate(x=w348) -> (-x=w337:dbl)
    n248 = Add(x=w337, y=0.3) -> (x+y=w338:dbl)
    n249 = Select(t=WPI_SolenoidValue."On" ("Value"), s=w376, f=WPI_SolenoidValue."Off" ("Value")) -> (s? t:f=w356:T26)
    n250 = call-poly <vilib>:"CTRE_Phoenix_MotorController_Get_Enhanced.vi"("PhoenixMotorControlDevRef"=w346) -> ("Quadrature Position"=w345:i32)  [unwired: 11 in, 3 out]
    n251 = call-poly <vilib>:"WPI_SolenoidSet.vi"("Value"=w356, "SolenoidDevRef"=w357) -> ()  [unwired: 8 in, 2 out]
    n252 = call-poly <vilib>:"WPI_SolenoidSet.vi"("Value"=w356, "SolenoidDevRef"=w379) -> ()  [unwired: 8 in, 2 out]
    n253 = Subtract(x=w345, y=w344) -> (x-y=w334:dbl)
    n254 = Greater Or Equal?(x=w334, y=w340) -> (x >= y?=w339:bool)
    n255 = Less Or Equal To 0?(x=w334) -> (x <= 0?=w335:bool)
    n256 = case shown="\"Fully Up\", Default" w343 {
      tunnel: w342 -> [w397 _ w412 _]
      tunnel: [w398 w399 w408 w414] -> w341
      tunnel: w339 -> [_ w402 _ _]
      tunnel: w338 -> [_ w401 _ _]
      tunnel: [0.0 w400 0.0 w413] -> w336
      tunnel: w335 -> [_ _ _ w415]
      frame "Fully Up", Default {
        n257 = Select(t=HAB_Bk_Spd_Motor_States."Going Down" ("HAB Bk Spd Motor States"), s=w397, f=HAB_Bk_Spd_Motor_States."Fully Up" ("HAB Bk Spd Motor States")) -> (s? t:f=w398:T12)
      }
      frame "Going Down" {
        n258 = case shown="True" w402 {
          tunnel: w401 -> [w404 _]
          tunnel: [w404 0.0] -> w400
          tunnel: [HAB_Bk_Spd_Motor_States."Going Down" ("HAB Bk Spd Motor States") HAB_Bk_Spd_Motor_States."Fully Down" ("HAB Bk Spd Motor States")] -> w399
          frame False {
          }
          frame True {
          }
        }
      }
      frame "Fully Down" {
        n259 = Not(x=w412) -> (.not. x?=w409:bool)
        n260 = Select(t=HAB_Bk_Spd_Motor_States."Going Up" ("HAB Bk Spd Motor States"), s=w409, f=HAB_Bk_Spd_Motor_States."Fully Down" ("HAB Bk Spd Motor States")) -> (s? t:f=w408:T12)
      }
      frame "Going Up" {
        n261 = case shown="True" w415 {
          tunnel: [-0.4 0.0] -> w413
          tunnel: [HAB_Bk_Spd_Motor_States."Going Up" ("HAB Bk Spd Motor States") HAB_Bk_Spd_Motor_States."Fully Up" ("HAB Bk Spd Motor States")] -> w414
          frame False {
            # "gently yeet the \nthing back up, but\nthe velocity don't\nmatter that much"
          }
          frame True {
          }
        }
      }
    }
    n262 = Select(t=WPI_SolenoidValue."On" ("Value"), s=w342, f=WPI_SolenoidValue."Off" ("Value")) -> (s? t:f=w375:T26)
    n263 = call-poly <vilib>:"WPI_SolenoidSet.vi"("Value"=w375, "SolenoidDevRef"=w372) -> ()  [unwired: 8 in, 2 out]
    n264 = Bundle By Name(cluster=w333, "HAB Bk Spd Motor States"=w341) -> (w332:T25)
    n265 = call <vilib>:"CTRE_Phoenix_MotorControl_Set.vi"("Output"=w336, "Control Mode"=w349, "PhoenixMotorControlDevRef"=w346) -> ()  [unwired: 7 in, 2 out]
    n266 = Unbundle By Name(w332) -> ("Front HAB 3 Limit Switch"=w371:T8)
    n267 = Unbundle By Name(w332) -> ("Back HAB 3 Limit Switch"=w369:T8)
    n268 = disable-structure shown="Disabled" {
      disable-tunnel: w332 -> [w497 _]
      frame Disabled {
        # "maybe use in range and coerce in future to\nprevent drivers from being able to drive\nthe module backwards?"
        # "slows down motor so\nwe don't damage the\ncylinders"
        n269 = Unbundle By Name(w497) -> ("Aux Joystick Indexes.Right Y"=w502:i32)
        n270 = Unbundle By Name(w497) -> ("HAB3DriveModuleMotorDevRef"=w504:T1)
        n271 = Unbundle By Name(w497) -> ("Aux Axes"=w503:dbl[])
        n272 = Index Array(array=w503, index=w502) -> (element=w499:dbl)
        n273 = call "Deadband.vi"("Input"=w499) -> ("Output"=w500:dbl)  [unwired: 10 in]
        n274 = Multiply(x=w500, y=0.3) -> (x*y=w498:dbl)
        n275 = call <vilib>:"WPI_MotorControlSetOutput.vi"("Output"=w498, "MotorControlDevRef"=w504) -> ()  [unwired: 7 in, 3 out]
      }
      frame Enabled {
      }
    }
    n276 = Unbundle By Name(w332) -> ("HAB3DriveModuleMotorDevRef"=w370:T1)
    n277 = Unbundle By Name(w332) -> ("Aux Joystick Indexes.Right Y"=w368:i32)
    n278 = Unbundle By Name(w332) -> ("Aux Axes"=w367:dbl[])
    n279 = call <vilib>:"WPI_DigitalInputGetValue.vi"("DigitalInputDevRef"=w369) -> ("Value"=w365:bool)  [unwired: 8 in, 2 out]
    n280 = call <vilib>:"WPI_DigitalInputGetValue.vi"("DigitalInputDevRef"=w371) -> ("Value"=w366:bool)  [unwired: 8 in, 2 out]
    n281 = Index Array(array=w367, index=w368) -> (element=w363:dbl)
    n282 = Not(x=w365) -> (.not. x?=w359:bool)
    n283 = Not(x=w366) -> (.not. x?=w360:bool)
    n284 = Or(x=w360, y=w359) -> (x .or. y?=w364:bool)
    n285 = case shown="False" w364 {
      tunnel: w370 -> [w512 w516]
      tunnel: w363 -> [w509 _]
      frame False {
        # "This is a range and coerce. :P \nSees if the joystick is going backwards.\n(If the value is negative).\nIf yes, then output is set to 0.\nIf no, then output is set from the aux\njoystick. \nWe don't want the robot to go \nbackwards off of the platform. LOL"
        # "Slows down the motor output\nso we don't damage the cylinders"
        n286 = call "Deadband.vi"("Input"=w509) -> ("Output"=w514:dbl)  [unwired: 10 in]
        n287 = In Range and Coerce(upper limit=0.0, x=w509, lower limit=-1.0) -> (In Range?=w508:bool)  [unwired: 1 out]
        n288 = Multiply(x=w514, y=0.3) -> (x*y=w507:dbl)
        n289 = Select(t=0.0, s=w508, f=w507) -> (s? t:f=w506:dbl)
        n290 = call <vilib>:"WPI_MotorControlSetOutput.vi"("Output"=w506, "MotorControlDevRef"=w512) -> ()  [unwired: 7 in, 3 out]
      }
      frame True {
        # "If either the \"Front HAB 3 Limit Switch\" or \"Front HAB 3 Limit Switch\"\nis pressed, the HAB 3 Drive Module set output will be \"0.\" \n- Preventing the DRIVER from moving too far forward into\nthe HAB 3 Platform, which can damage the cylinders.\n\nIf not, the aux joysick will control the set output.\n- Enabling the DRIVER to drive forward until the robot reaches the\nplatform"
        n291 = call <vilib>:"WPI_MotorControlSetOutput.vi"("Output"=0.0, "MotorControlDevRef"=w516) -> ()  [unwired: 7 in, 3 out]
      }
    }
  }
  n292 = while {
    shift-right: [w637] -> _
    shift-left: w108 -> [w624]
    tunnel: w29 -> [w598]
    stop <- FALSE stop-if-true
    # "0 = Side-by-side stream\n1 = The secondary camera is placed\n       in the lower-right corner\n2 = The primary camera stream is\n       placed in the lower-right corner"
    # "converts encoder values\nto inches for auto if necessary"
    # "Parse our motion profile csv, each row is a trajectory point"
    # "Parse our motion profile csv, each row is a trajectory point"
    # "this allows us to exit the MP \neither if it finishes (since the\nMP control VI makes the\nlatch false when finished) \nor by pressing the cancel \nbutton"
    # "these numbers are the indexes of\nthe drive motors based on the\norder that they're opened in Begin"
    # "the Ys of the drive joysticks are \ninverted by default"
    n293 = disable-structure shown="Disabled" {
      disable-tunnel: w598 -> [w806 _]
      frame Disabled {
        n294 = call <vilib>:"WPI_GyroGetAngle.vi"("GyroDevRef"=w806) -> ("Angle"=w807:dbl)  [unwired: 6 in, 4 out]
        n295 = global write "Robot Global Data.vi" "Gyro"(w807) -> ()
      }
      frame Enabled {
      }
    }
    n296 = Unbundle By Name(w624) -> ("DriveJoystickDevRef"=w635:T9)
    n297 = Unbundle By Name(w624) -> ("AuxJoystickDevRef"=w634:T9)
    n298 = Unbundle By Name(w624) -> ("Robot Mode"=w633:T16)
    n299 = call <vilib>:"WPI_JoystickGetValues.vi"("JoystickDevRef"=w634) -> ("Buttons"=w626:bool[], "Axes"=w627:dbl[], "JoystickDevRef"=w628:T9, "POVs"=w625:i16[])  [unwired: 6 in, 1 out]
    n300 = call <vilib>:"WPI_JoystickGetValues.vi"("JoystickDevRef"=w635) -> ("Buttons"=w630:bool[], "Axes"=w632:dbl[], "JoystickDevRef"=w631:T9, "POVs"=w629:i16[])  [unwired: 6 in, 1 out]
    n301 = case shown="\"Teleop Enabled\"" w633 {
      tunnel: w624 -> [w820 w836 w838 w854 w856 w863 w872 w888 w890]
      tunnel: [w819 w827 w837 w845 w855 w864 w871 w879 w889] -> w597
      tunnel: w632 -> [_ w835 _ w852 _ _ _ w886 _]
      tunnel: w631 -> [_ w834 _ w853 _ _ _ w887 _]
      tunnel: w630 -> [_ w833 _ w851 _ _ _ w885 _]
      tunnel: w629 -> [_ w832 _ w850 _ _ _ w884 _]
      tunnel: w628 -> [_ w831 _ w849 _ _ _ w883 _]
      tunnel: w627 -> [_ w830 _ w848 _ _ _ w882 _]
      tunnel: w626 -> [_ w829 _ w847 _ _ _ w881 _]
      tunnel: w625 -> [_ w828 _ w846 _ _ _ w880 _]
      frame "Autonomous Disabled", Default {
        n302 = disable-structure shown="Enabled" {
          disable-tunnel: w820 -> [w822 w826]
          disable-tunnel: [w821 w825] -> w819
          frame Disabled {
            n303 = Bundle By Name(cluster=w822, "Joystick VS Vision Latch"=FALSE) -> (w821:T23)
          }
          frame Enabled {
            n304 = Bundle By Name(cluster=w826, "Vision States"=Vision_States."Ready") -> (w825:T23)
          }
        }
      }
      frame "Autonomous Enabled" {
        n305 = Bundle By Name(cluster=w836, "DriveJoystickDevRef"=w834, "Drive Axes"=w835, "Drive Buttons"=w833, "Drive POVs"=w832, "AuxJoystickDevRef"=w831, "Aux Axes"=w830, "Aux Buttons"=w829, "Aux POVs"=w828) -> (w827:T23)
      }
      frame "Teleop Disabled" {
        n306 = disable-structure shown="Enabled" {
          disable-tunnel: w838 -> [w840 w844]
          disable-tunnel: [w839 w843] -> w837
          frame Disabled {
            n307 = Bundle By Name(cluster=w840, "Joystick VS Vision Latch"=FALSE) -> (w839:T23)
          }
          frame Enabled {
            n308 = Bundle By Name(cluster=w844, "Vision States"=Vision_States."Ready") -> (w843:T23)
          }
        }
      }
      frame "Teleop Enabled" {
        n309 = Bundle By Name(cluster=w854, "DriveJoystickDevRef"=w853, "Drive Axes"=w852, "Drive Buttons"=w851, "Drive POVs"=w850, "AuxJoystickDevRef"=w849, "Aux Axes"=w848, "Aux Buttons"=w847, "Aux POVs"=w846) -> (w845:T23)
      }
      frame "Disconnected" {
        n310 = disable-structure shown="Enabled" {
          disable-tunnel: w856 -> [w858 w862]
          disable-tunnel: [w857 w861] -> w855
          frame Disabled {
            n311 = Bundle By Name(cluster=w858, "Joystick VS Vision Latch"=FALSE) -> (w857:T23)
          }
          frame Enabled {
            n312 = Bundle By Name(cluster=w862, "Vision States"=Vision_States."Ready") -> (w861:T23)
          }
        }
      }
      frame "Finish" {
        n313 = disable-structure shown="Enabled" {
          disable-tunnel: w863 -> [w866 w870]
          disable-tunnel: [w865 w869] -> w864
          frame Disabled {
            n314 = Bundle By Name(cluster=w866, "Joystick VS Vision Latch"=FALSE) -> (w865:T23)
          }
          frame Enabled {
            n315 = Bundle By Name(cluster=w870, "Vision States"=Vision_States."Ready") -> (w869:T23)
          }
        }
      }
      frame "Test Disabled" {
        n316 = disable-structure shown="Enabled" {
          disable-tunnel: w872 -> [w874 w878]
          disable-tunnel: [w873 w877] -> w871
          frame Disabled {
            n317 = Bundle By Name(cluster=w874, "Joystick VS Vision Latch"=FALSE) -> (w873:T23)
          }
          frame Enabled {
            n318 = Bundle By Name(cluster=w878, "Vision States"=Vision_States."Ready") -> (w877:T23)
          }
        }
      }
      frame "Test Enabled" {
        n319 = Bundle By Name(cluster=w888, "DriveJoystickDevRef"=w887, "Drive Axes"=w886, "Drive Buttons"=w885, "Drive POVs"=w884, "AuxJoystickDevRef"=w883, "Aux Axes"=w882, "Aux Buttons"=w881, "Aux POVs"=w880) -> (w879:T23)
      }
      frame "Emergency Stopped" {
        n320 = disable-structure shown="Enabled" {
          disable-tunnel: w890 -> [w892 w896]
          disable-tunnel: [w891 w895] -> w889
          frame Disabled {
            n321 = Bundle By Name(cluster=w892, "Joystick VS Vision Latch"=FALSE) -> (w891:T23)
          }
          frame Enabled {
            n322 = Bundle By Name(cluster=w896, "Vision States"=Vision_States."Ready") -> (w895:T23)
          }
        }
      }
    }
    n323 = Wait (ms)(milliseconds to wait=u32 50) -> ()  [unwired: 1 out]
    n324 = call-poly <vilib>:"NT Write Value.vi"("Numeric"=2, "Name"="/limelight/stream") -> ()  [unwired: 9 in, 1 out]
    n325 = Unbundle By Name(w597) -> ("Drive Joystick Indexes.Left X"=w605:i32, "Drive Joystick Indexes.Left Y"=w606:i32, "Drive Joystick Indexes.Right X"=w607:i32, "Drive Joystick Indexes.Right Y"=w608:i32)
    n326 = Unbundle By Name(w597) -> ("Drive Motors.Motors[]"=w596:T1[])
    n327 = Unbundle By Name(w597) -> ("Drive Buttons"=w603:bool[])
    n328 = Unbundle By Name(w597) -> ("Drive Button Indexes.A Button"=w620:i32)
    n329 = Unbundle By Name(w597) -> ("Drive Buttons"=w602:bool[])
    n330 = Unbundle By Name(w597) -> ("Drive Button Indexes.LB Button"=w601:i32)
    n331 = Unbundle By Name(w597) -> ("Joystick VS Vision Latch"=w622:bool)
    n332 = Unbundle By Name(w597) -> ("Drive Axes"=w604:dbl[])
    n333 = global read "Robot Global Data.vi" "Robot Mode"() -> (w609:T16)
    n334 = Index Array(array=w596, index #1=2 ("index"), index #2=3 ("index")) -> (element #1=w595:T1, element #2=w594:T1)
    n335 = Bundle By Name(cluster=w597, "Robot Mode"=w609) -> (w623:T23)
    n336 = Index Array(array=w603, index=w620) -> (element=w621:bool)
    n337 = global read "Robot Global Data.vi" "Which Robot?"() -> (w560:T28)
    n338 = Index Array(array=w604, index #1=w605, index #2=w606, index #3=w607, index #4=w608) -> (element #1=w613:dbl, element #2=w614:dbl, element #3=w615:dbl, element #4=w616:dbl)
    n339 = global read "Robot Global Data.vi" "Which Robot?"() -> (w566:T28)
    n340 = Index Array(array=w602, index=w601) -> (element=w599:bool)
    n341 = global read "Robot Global Data.vi" "Right Encoder Val. Initial"() -> (w567:dbl)
    n342 = global read "Robot Global Data.vi" "Left Encoder Val. Initial"() -> (w569:dbl)
    n343 = disable-structure shown="Enabled" {
      disable-tunnel: w621 -> [w810 w817]
      disable-tunnel: w622 -> [_ w815]
      disable-tunnel: w623 -> [_ w813]
      disable-tunnel: [_ w811] -> w600
      frame Disabled {
        n344 = feedback #9() -> (w809:bool)  [unwired: 1 in]
        n345 = feedback-in #9(w810) -> ()
        n346 = Greater?(x=w810, y=w809) -> (0:w808:bool)
        n347 = global write "Robot Global Data.vi" "Driver VS Vision Control"(w808) -> ()
      }
      frame Enabled {
        n348 = feedback #10() -> (w818:bool)  [unwired: 1 in]
        n349 = feedback-in #10(w817) -> ()
        n350 = Greater?(x=w817, y=w818) -> (0:w816:bool)
        n351 = Not(x=w815) -> (.not. x?=w814:bool)
        n352 = Select(t=w814, s=w816, f=w815) -> (s? t:f=w812:bool)
        n353 = global write "Robot Global Data.vi" "Driver VS Vision Control"(w812) -> ()
        n354 = Bundle By Name(cluster=w813, "Joystick VS Vision Latch"=w812) -> (w811:T23)
      }
    }
    n355 = call "Deadband.vi"("Input"=w613) -> ("Output"=w611:dbl)  [unwired: 10 in]
    n356 = call "Deadband.vi"("Input"=w614) -> ("Output"=w612:dbl)  [unwired: 10 in]
    n357 = call "Deadband.vi"("Input"=w615) -> ("Output"=w610:dbl)  [unwired: 10 in]
    n358 = call "Deadband.vi"("Input"=w616) -> ("Output"=w617:dbl)  [unwired: 10 in]
    n359 = call-poly <vilib>:"CTRE_Phoenix_MotorController_Get_Enhanced.vi"("PhoenixMotorControlDevRef"=w595) -> ("Quadrature Position"=w570:i32)  [unwired: 11 in, 3 out]
    n360 = call-poly <vilib>:"CTRE_Phoenix_MotorController_Get_Enhanced.vi"("PhoenixMotorControlDevRef"=w594) -> ("Quadrature Position"=w568:i32)  [unwired: 11 in, 3 out]
    n361 = Negate(x=w612) -> (-x=w618:dbl)
    n362 = Negate(x=w617) -> (-x=w619:dbl)
    n363 = global write "Robot Global Data.vi" "Left Drive Joystick X"(w611) -> ()
    n364 = global write "Robot Global Data.vi" "Right Drive Joystick X"(w610) -> ()
    n365 = case shown="\"Competition Bot\", Default" w560 {
      tunnel: [w640 w642 w644] -> w559
      tunnel: [w639 w641 w643] -> w558
      frame "Competition Bot", Default {
        w639 = 18069  # Change in Encoder
        w640 = 84  # Change in Distance (inches)
      }
      frame "Practice Bot" {
        w641 = 0  # Change in Encoder
        w642 = 0  # Change in Distance (inches)
      }
      frame "Code Bot" {
        w643 = 0  # Change in Encoder
        w644 = 0  # Change in Distance (inches)
      }
    }
    n366 = global write "Robot Global Data.vi" "Right Drive Joystick Y"(w619) -> ()
    n367 = global write "Robot Global Data.vi" "Left Drive Joystick Y"(w618) -> ()
    n368 = case shown="\"Competition Bot\", Default" w566 {
      tunnel: [w646 w648 w650] -> w565
      tunnel: [w645 w647 w649] -> w564
      frame "Competition Bot", Default {
        w645 = 17996  # Change in Encoder
        w646 = 84  # Change in Distance (inches)
      }
      frame "Practice Bot" {
        w647 = 0  # Change in Encoder
        w648 = 0  # Change in Distance (inches)
      }
      frame "Code Bot" {
        w649 = 0  # Change in Encoder
        w650 = 0  # Change in Distance (inches)
      }
    }
    n369 = Subtract(x=w570, y=w569) -> (x-y=w562:dbl)
    n370 = Subtract(x=w568, y=w567) -> (x-y=w556:dbl)
    n371 = Bundle By Name(cluster=w600, "Vision Track Mode Override"=w599) -> (w588:T23)
    n372 = global write "Robot Global Data.vi" "Right Encoder in Enc. Vals"(w556) -> ()
    n373 = global write "Robot Global Data.vi" "Left Encoder in Enc. Vals"(w562) -> ()
    n374 = Divide(x=w559, y=w558) -> (x/y=w555:dbl)
    n375 = Divide(x=w565, y=w564) -> (x/y=w563:dbl)
    n376 = Multiply(x=w563, y=w562) -> (x*y=w561:dbl)
    n377 = Multiply(x=w556, y=w555) -> (x*y=w557:dbl)
    n378 = global write "Robot Global Data.vi" "Left Encoder in Inches"(w561) -> ()
    n379 = global write "Robot Global Data.vi" "Right Encoder in Inches"(w557) -> ()
    n380 = disable-structure shown="Enabled" {
      disable-tunnel: w588 -> [w700 w707]
      frame Disabled {
        n381 = Unbundle By Name(w700) -> ("Drive Button Indexes.RB Button"=w699:i32)
        n382 = Unbundle By Name(w700) -> ("Drive Buttons"=w698:bool[])
        n383 = Unbundle By Name(w700) -> ("T = Motion Profile, F = Percent Output"=w693:bool)
        n384 = Index Array(array=w698, index=w699) -> (element=w696:bool)
        n385 = feedback #11() -> (w697:bool)  [unwired: 1 in]
        n386 = feedback-in #11(w696) -> ()
        n387 = Greater?(x=w696, y=w697) -> (0:w695:bool)
        n388 = Not(x=w693) -> (.not. x?=w694:bool)
        n389 = Select(t=w694, s=w695, f=w693) -> ()  [unwired: 1 out]
      }
      frame Enabled {
        n390 = Unbundle By Name(w707) -> ("Drive Button Indexes.RB Button"=w709:i32)
        n391 = Unbundle By Name(w707) -> ("Drive Buttons"=w708:bool[])
        n392 = global read "Robot Global Data.vi" "Cancel the Motion Profile?"() -> (w701:bool)
        n393 = Index Array(array=w708, index=w709) -> (element=w703:bool)
        n394 = feedback #12() -> (w706:bool)  [unwired: 1 in]
        n395 = feedback-in #12(w703) -> ()
        n396 = Greater?(x=w703, y=w706) -> (0:w705:bool)
        n397 = Not(x=w701) -> (.not. x?=w704:bool)
        n398 = Select(t=w704, s=w705, f=w701) -> (s? t:f=w702:bool)
        n399 = global write "Robot Global Data.vi" "Cancel the Motion Profile?"(w702) -> ()
      }
    }
    n400 = Unbundle By Name(w588) -> ("T = Motion Profile, F = Percent Output"=w585:bool)
    n401 = global read "Robot Global Data.vi" "Run the Motion Profile?"() -> (w587:bool)
    n402 = And(x=w587, y=w585) -> (x .and. y?=w586:bool)
    n403 = Bundle By Name(cluster=w588, "T = Motion Profile, F = Percent Output"=w586) -> (w591:T23)
    n404 = call "RIGHT Motion Profile Traj Points Array.vi"("Read = false, Write = true"=FALSE) -> ("traj. points array out"=w571:dbl[][])  [unwired: 10 in]
    "Right Traj. Pts Array" <- w571
    n405 = call "LEFT Motion Profile Traj Points Array.vi"("Read = false, Write = true"=FALSE) -> ("traj. points array out"=w578:dbl[][])  [unwired: 10 in]
    "Left Traj. Pts Array" <- w578
    n406 = for {
      N -> [w664]
      tunnel: w571 -> [w670] mode=indexing
      tunnel: [w660] -> w577 mode=indexing
      i -> [w663]
      w669 = 0.0 ("Arbitrary Feed Forward")
      # "Convert profile units to talon units"
      n407 = Decrement(x=w664) -> (x-1=w665:i32)
      n408 = Equal?(x=w665, y=w663) -> (x = y?=w666:bool)
      n409 = Equal To 0?(x=w663) -> (x = 0?=w662:bool)
      n410 = Index Array(array=w670) -> (element #1=w658:dbl, element #2=w652:dbl, element #3=w659:dbl)  [unwired: 3 in]
      n411 = Multiply(x=4096.0, y=w652) -> (x*y=w654:dbl)
      n412 = Multiply(x=4096.0, y=w658) -> (x*y=w656:dbl)
      n413 = Divide(x=w654, y=10.0) -> (x/y=w651:dbl)
      n414 = Bundle By Name(cluster=T31 {"Position"=0.0, "Velocity"=0.0, "Arbitrary Feed Forward"=0.0, "Auxiliary Position"=0.0, "Auxiliary Velocity"=0.0, "Auxiliary Arbitrary Feed Forward"=0.0, "Profile Slot Select"=0, "Auxiliary Profile Slot Select"=0, "isLastPoint?"=FALSE, "Zero Position?"=FALSE, "durationMs"=0, "Use Aux PID?"=FALSE} ("Trajectory Point"), "Position"=w656, "Velocity"=w651, "Arbitrary Feed Forward"=w669, "Auxiliary Position"=w669, "Auxiliary Velocity"=w669, "Auxiliary Arbitrary Feed Forward"=w669, "Profile Slot Select"=0, "Auxiliary Profile Slot Select"=1, "isLastPoint?"=w666, "Zero Position?"=w662, "durationMs"=w659, "Use Aux PID?"=FALSE) -> (w660:T31)
    }
    n415 = for {
      N -> [w685]
      tunnel: w578 -> [w691] mode=indexing
      tunnel: [w681] -> w584 mode=indexing
      i -> [w684]
      w690 = 0.0 ("Arbitrary Feed Forward")
      # "Convert profile units to talon units"
      n416 = Decrement(x=w685) -> (x-1=w686:i32)
      n417 = Equal?(x=w686, y=w684) -> (x = y?=w687:bool)
      n418 = Equal To 0?(x=w684) -> (x = 0?=w683:bool)
      n419 = Index Array(array=w691) -> (element #1=w679:dbl, element #2=w673:dbl, element #3=w680:dbl)  [unwired: 3 in]
      n420 = Multiply(x=4096.0, y=w673) -> (x*y=w675:dbl)
      n421 = Multiply(x=4096.0, y=w679) -> (x*y=w677:dbl)
      n422 = Divide(x=w675, y=10.0) -> (x/y=w672:dbl)
      n423 = Bundle By Name(cluster=T31 {"Position"=0.0, "Velocity"=0.0, "Arbitrary Feed Forward"=0.0, "Auxiliary Position"=0.0, "Auxiliary Velocity"=0.0, "Auxiliary Arbitrary Feed Forward"=0.0, "Profile Slot Select"=0, "Auxiliary Profile Slot Select"=0, "isLastPoint?"=FALSE, "Zero Position?"=FALSE, "durationMs"=0, "Use Aux PID?"=FALSE} ("Trajectory Point"), "Position"=w677, "Velocity"=w672, "Arbitrary Feed Forward"=w690, "Auxiliary Position"=w690, "Auxiliary Velocity"=w690, "Auxiliary Arbitrary Feed Forward"=w690, "Profile Slot Select"=0, "Auxiliary Profile Slot Select"=1, "isLastPoint?"=w687, "Zero Position?"=w683, "durationMs"=w680, "Use Aux PID?"=FALSE) -> (w681:T31)
    }
    n424 = call <vilib>:"CTRE_Phoenix_MotorControl_BufferedTrajectoryPointStream_Open.vi"() -> ("BufferedTrajectoryPointStream_DevRef"=w576:T32)  [unwired: 10 in, 1 out]
    n425 = call <vilib>:"CTRE_Phoenix_MotorControl_BufferedTrajectoryPointStream_Open.vi"() -> ("BufferedTrajectoryPointStream_DevRef"=w583:T32)  [unwired: 10 in, 1 out]
    n426 = call-poly <vilib>:"CTRE_Phoenix_MotorControl_BufferedTrajectoryPointStream_Write.vi"("Motion Profile Trajectory Point Array"=w577, "BufferedTrajectoryPointStream_DevRef"=w576) -> ("error out"=w574:errorcluster, "BufferedTrajectoryPointStream_DevRef"=w575:T32)  [unwired: 8 in]
    n427 = call-poly <vilib>:"CTRE_Phoenix_MotorControl_BufferedTrajectoryPointStream_Write.vi"("Motion Profile Trajectory Point Array"=w584, "BufferedTrajectoryPointStream_DevRef"=w583) -> ("error out"=w581:errorcluster, "BufferedTrajectoryPointStream_DevRef"=w582:T32)  [unwired: 8 in]
    n428 = call <vilib>:"CTRE_Phoenix_MotorControl_BufferedTrajectoryPointStream_SetDeviceReference.vi"("error in (no error)"=w574, "refnum name"="right_mpStream", "BufferedTrajectoryPointStream_DevRef"=w575) -> ()  [unwired: 7 in, 2 out]
    n429 = call <vilib>:"CTRE_Phoenix_MotorControl_BufferedTrajectoryPointStream_SetDeviceReference.vi"("error in (no error)"=w581, "refnum name"="left_mpStream", "BufferedTrajectoryPointStream_DevRef"=w582) -> ()  [unwired: 7 in, 2 out]
    n430 = Unbundle By Name(w591) -> ("T = Motion Profile, F = Percent Output"=w590:bool)
    n431 = feedback-in #13(w590) -> ()
    n432 = feedback #13() -> (w589:bool)  [unwired: 1 in]
    n433 = case shown="True" w590 {
      selector: w590 -> [_ w805]
      tunnel: [w711 w802] -> w637
      tunnel: w591 -> [w710 w803]
      tunnel: w589 -> [_ w804]
      frame False {
        n434 = disable-structure shown="Enabled" {
          disable-tunnel: [w727 w746] -> w711
          disable-tunnel: w710 -> [w719 w732]
          frame Enabled {
            # "Vision and Joystick Control for Drive Train"
            # "for ease of testing\nfor programmers"
            # "1 = force off\n3 = force on"
            # "0 = vision processor\n1 = driver camera settings"
            n435 = Unbundle By Name(w719) -> ("Joystick VS Vision Latch"=w723:bool)
            n436 = Unbundle By Name(w719) -> ("Vision Track Mode Override"=w715:bool)
            n437 = Select(t=3, s=w723, f=1) -> (s? t:f=w714:i32)
            n438 = Select(t=0, s=w723, f=1) -> (s? t:f=w718:i32)
            n439 = Select(t=3, s=w715, f=w714) -> (s? t:f=w713:i32)
            n440 = Select(t=0, s=w715, f=w718) -> (s? t:f=w716:i32)
            n441 = case shown="False" w723 {
              tunnel: w719 -> [w728 w730]
              tunnel: [w728 w729] -> w727
              frame False {
                n442 = call "Joystick Drive Control.vi"("Cluster"=w728) -> ()  [unwired: 11 in]
              }
              frame True {
                n443 = call "Vision Tracking Drive Control.vi"("Cluster in"=w730) -> ("Cluster out"=w729:T33)  [unwired: 10 in]
              }
            }
            n444 = call-poly <vilib>:"NT Write Value.vi"("Numeric"=w716, "Name"="/limelight/camMode") -> ()  [unwired: 9 in, 1 out]
            n445 = call-poly <vilib>:"NT Write Value.vi"("Numeric"=w713, "Name"="/limelight/ledMode") -> ()  [unwired: 9 in, 1 out]
          }
          frame Disabled {
            n446 = call-poly <vilib>:"NT Read Value.vi"("Name"="/limelight/tx") -> ("Numeric"=w740:dbl)  [unwired: 9 in, 1 out]
            n447 = call-poly <vilib>:"NT Read Value.vi"("Name"="/limelight/ty") -> ("Numeric"=w739:dbl)  [unwired: 9 in, 1 out]
            n448 = call-poly <vilib>:"NT Read Value.vi"("Name"="/limelight/ta") -> ("Numeric"=w738:dbl)  [unwired: 9 in, 1 out]
            n449 = call-poly <vilib>:"NT Read Value.vi"("Name"="/limelight/ts") -> ("Numeric"=w737:dbl)  [unwired: 9 in, 1 out]
            n450 = call-poly <vilib>:"NT Read Value.vi"("Name"="/limelight/tshort") -> ("Numeric"=w734:dbl)  [unwired: 9 in, 1 out]
            n451 = call-poly <vilib>:"NT Read Value.vi"("Name"="/limelight/tlong") -> ("Numeric"=w733:dbl)  [unwired: 9 in, 1 out]
            n452 = Bundle By Name(cluster=w732, "limelight.offsetAngle H"=w740, "limelight.offsetAngle V"=w739, "limelight.area"=w738, "limelight.skew"=w737, "limelight.shortest side (pxls)"=w734, "limelight.longest side (pxls)"=w733) -> (w731:T23)
            n453 = Unbundle By Name(w731) -> ("Vision States"=w748:T18)
            n454 = case shown="\"Ready\", Default" w748 {
              tunnel: [w749 w764 w782] -> w747
              tunnel: w731 -> [w749 w764 w782]
              tunnel: [w758 w765 w778] -> w745
              frame "Ready", Default {
                # "should have created a \nboolean in the cluster \ninstead of just pulling\nthe A button"
                # "the Ys of the drive joysticks are \ninverted by default"
                n455 = Unbundle By Name(w749) -> ("Drive Button Indexes.A Button"=w763:i32)
                n456 = Unbundle By Name(w749) -> ("Drive Buttons"=w762:bool[])
                n457 = Unbundle By Name(w749) -> ("Drive Motors"=w757:T11, "Drive Axes"=w756:dbl[], "Drive Joystick Indexes.Left Y"=w755:i32, "Drive Joystick Indexes.Right Y"=w754:i32)
                n458 = Index Array(array=w762, index=w763) -> (element=w761:bool)
                n459 = Index Array(array=w756, index #1=w755, index #2=w754) -> (element #1=w753:dbl, element #2=w752:dbl)
                n460 = Negate(x=w753) -> (-x=w750:dbl)
                n461 = Negate(x=w752) -> (-x=w751:dbl)
                n462 = Select(t=Vision_States."Forward Until Target at Edge" ("Vision States"), s=w761, f=Vision_States."Ready" ("Vision States")) -> (s? t:f=w758:T18)
                n463 = call <vilib>:"WPI_RobotDriveTankDrive.vi"("Right axis value"=w751, "Left axis value"=w750, "RobotDriveDevRef"=w757) -> ()  [unwired: 6 in, 3 out]
              }
              frame "Forward Until Target at Edge" {
                n464 = Unbundle By Name(w764) -> ("limelight.offsetAngle H"=w769:dbl)
                n465 = Less?(x=w769, y=-26) -> (x < y?=w767:bool)
                n466 = Greater?(x=w769, y=14) -> (0:w768:bool)
                n467 = Or(x=w768, y=w767) -> (x .or. y?=w766:bool)
                n468 = case shown="False" w766 {
                  tunnel: [Vision_States."Forward Until Target at Edge" ("Vision States") Vision_States."Vision Track" ("Vision States")] -> w765
                  tunnel: w764 -> [w775 _]
                  frame False {
                    w773 = 0.35
                    n469 = Unbundle By Name(w775) -> ("Drive Motors"=w774:T11)
                    n470 = call <vilib>:"WPI_RobotDriveTankDrive.vi"("Right axis value"=w773, "Left axis value"=w773, "RobotDriveDevRef"=w774) -> ()  [unwired: 6 in, 3 out]
                  }
                  frame True {
                  }
                }
              }
              frame "Vision Track" {
                w785 = 0.5 ("t")
                w784 = 1.5
                # "this is the target area for\nwhen to stop driving \ntoward target (10 here \nwould means 10% of \nlimelight feed)"
                # "Hori. offset scaled down to\nbe a reasonable drive speed\ncoefficient (e.g. if this number\nis 0.01, 10deg offset to the \nleft would make right train \nrun at 110% and left train \nat 90%)"
                # "0deg offset = speed \nadjustment coefficient of 1"
                n471 = Unbundle By Name(w782) -> ("limelight.area"=w790:dbl, "limelight.offsetAngle H"=w798:dbl)
                n472 = Multiply(x=w798, y=0.03) -> (x*y=w787:dbl)
                n473 = Unbundle By Name(w782) -> ("Drive Motors"=w783:T11)
                n474 = Add(x=1.0, y=w787) -> (x+y=w793:dbl)
                n475 = Subtract(x=1.0, y=w787) -> (x-y=w786:dbl)
                n476 = Less?(x=w790, y=w784) -> (x < y?=w781:bool)
                n477 = Less?(x=w790, y=w784) -> (x < y?=w794:bool)
                n478 = Select(t=w785, s=w781, f=0.0) -> (s? t:f=w799:dbl)
                n479 = Select(t=w785, s=w794, f=0.0) -> (s? t:f=w791:dbl)
                n480 = Multiply(x=w799, y=w793) -> (x*y=w796:dbl)
                n481 = Multiply(x=w786, y=w791) -> (x*y=w789:dbl)
                n482 = Not(x=w781) -> (.not. x?=w777:bool)
                n483 = call <vilib>:"WPI_RobotDriveTankDrive.vi"("Right axis value"=w789, "Left axis value"=w796, "RobotDriveDevRef"=w783) -> ()  [unwired: 6 in, 3 out]
                n484 = Select(t=Vision_States."Ready" ("Vision States"), s=w777, f=Vision_States."Vision Track" ("Vision States")) -> (s? t:f=w778:T18)
              }
            }
            n485 = Bundle By Name(cluster=w747, "Vision States"=w745) -> (w746:T23)
          }
        }
      }
      frame True {
        # "left MP will control when the motion profile ends"
        # "Motion Profile Control for Drive Train"
        n486 = Greater?(x=w805, y=w804) -> (0:w801:bool)
        n487 = call "Motion Profile Left Drive Control.vi"("Start Motion Profile?"=w801, "Cluster in"=w803) -> ("Cluster out"=w802:T33)  [unwired: 9 in]
        n488 = call "Motion Profile Right Drive Control.vi"("Start Motion Profile?"=w801, "Cluster in"=w803) -> ()  [unwired: 9 in, 1 out]
      }
    }
  }
  n489 = disable-structure shown="Enabled" {
    frame Disabled {
      # "collector \nangle \nup/down"
      # "HAB 3 drive\nmodule"
      # "RJ"
      # "LJ"
      # "angle preset hover\nfor dust pan"
      # "angle preset out/down"
      # "angle preset in/up"
      # "lift hatch"
      # "retain hatch"
      # "kick hatch"
      # "RB"
      # "RT"
      # "LB"
      # "LT"
      # "back cylinders only"
      # "both cylinders"
      # "front cylinders only"
      # "x"
      # "a"
      # "b"
      # "y"
    }
    frame Disabled {
      # "inaccurate"
      # "collector \nangle \nup/down."
      # "HAB 3 drive\nmodule."
      # "RJ"
      # "LJ"
      # "angle preset hover\nfor dust pan."
      # "angle preset out/down"
      # "angle preset in/up."
      # "lift hatch."
      # "retain hatch."
      # "kick hatch."
      # "RB"
      # "RT"
      # "LB"
      # "LT"
      # "back cylinders only."
      # "both cylinders."
      # "front cylinders only."
      # "x"
      # "a"
      # "b"
      # "y"
    }
    frame Enabled {
    }
  }
  n490 = call "Reset Drive Encoders.vi"() -> ()  [unwired: 12 in]
  "error out" <- "error in"
